vi "filter pipe - complex.vi"(0 "omega  in":dbl[](array[numeric]), 2 "z in":cdb[](array[numeric]), 3 "delta":dbl=0.07, 5 "span":dbl=0.01, 6 "init":bool, 7 "interpolated gamma (kHz)":dbl, 8 "step once":bool, 9 "filter method":T1) -> (10 "center":cdb=0.005233304275841307+0.002092688467219436i, 12 "norm":dbl=0.0018669991905548619, 13 "at right end?":bool=TRUE, 14 "omega out":dbl[](array[numeric])=[2475.05, 2475.14, 2475.23, 2475.32, 2475.41, 2475.5, 2475.59, 2475.68, 2475.77, 2475.86, 2475.95, 2476.04, 2476.13, 2476.22, 2476.31, 2476.4, 2476.49, 2476.58, 2476.67, 2476.76, 2476.85, 2476.94, 2477.03, 2477.12, 2477.21, 2477.3, 2477.39, 2477.48, 2477.57, 2477.66, 2477.75, 2477.84, 2477.93, 2478.02, 2478.11, 2478.2, 2478.29, 2478.38, 2478.47, 2478.56, 2478.65, 2478.74, 2478.83, 2478.92, 2479.01, 2479.1, 2479.19, 2479.28, 2479.37, 2479.46, 2479.55, 2479.64, 2479.73, 2479.82, 2479.91, 2480.0, 2480.09, 2480.18, 2480.27, 2480.36, 2480.45, 2480.54, 2480.63, 2480.72, 2480.81, 2480.9, 2480.99, 2481.08, 2481.17, 2481.26, 2481.35, 2481.44, 2481.53, 2481.62, 2481.71, 2481.8, 2481.89, 2481.98, 2482.07, 2482.16, 2482.25, 2482.34, 2482.43, 2482.52, 2482.61, 2482.7, 2482.79, 2482.88, 2482.97, 2483.06, 2483.15, 2483.24, 2483.33, 2483.42, 2483.51, 2483.6, 2483.69, 2483.78, 2483.87, 2483.96, 2484.05, 2484.14, 2484.23, 2484.32, 2484.41, 2484.5, 2484.59, 2484.68, 2484.77, 2484.86, 2484.95, 2485.04, 2485.13, 2485.22, 2485.31, 2485.4, 2485.49, 2485.58, 2485.67, 2485.76, 2485.85, 2485.94, 2486.03, 2486.12, 2486.21, 2486.3, 2486.39, 2486.48, 2486.57, 2486.66, 2486.75, 2486.84, 2486.93, 2487.02, 2487.11, 2487.2, 2487.29, 2487.38, 2487.47, 2487.56, 2487.65, 2487.74, 2487.83, 2487.92, 2488.01, 2488.1, 2488.19, 2488.28, 2488.37, 2488.46, 2488.55, 2488.64, 2488.73, 2488.82, 2488.91, 2489.0, 2489.09, 2489.18, 2489.27, 2489.36, 2489.45, 2489.54, 2489.63, 2489.72, 2489.81, 2489.9, 2489.99, 2490.08, 2490.17, 2490.26, 2490.35, 2490.44, 2490.53, 2490.62, 2490.71, 2490.8, 2490.89, 2490.98, 2491.07, 2491.16, 2491.25, 2491.34, 2491.43, 2491.52, 2491.61, 2491.7, 2491.79, 2491.88, 2491.97, 2492.06, 2492.15, 2492.24, 2492.33, 2492.42, 2492.51, 2492.6, 2492.69, 2492.78, 2492.87, 2492.96, 2493.05, 2493.14, 2493.23, 2493.32, 2493.41, 2493.5, 2493.59, 2493.68, 2493.77, 2493.86, 2493.95, 2494.04, 2494.13, 2494.22, 2494.31, 2494.4, 2494.49, 2494.58, 2494.67, 2494.76, 2494.85, 2494.94, 2495.03, 2495.12, 2495.21, 2495.3, 2495.39, 2495.48, 2495.57, 2495.66, 2495.75, 2495.84, 2495.93, 2496.02, 2496.11, 2496.2, 2496.29, 2496.38, 2496.47, 2496.56, 2496.65, 2496.74, 2496.83, 2496.92, 2497.01, 2497.1, 2497.19, 2497.28, 2497.37, 2497.46, 2497.55, 2497.64, 2497.73, 2497.82, 2497.91, 2498.0, 2498.09, 2498.18, 2498.27, 2498.36, 2498.45, 2498.54, 2498.63, 2498.72, 2498.81, 2498.9, 2498.99, 2499.08, 2499.17, 2499.26, 2499.35, 2499.44, 2499.53, 2499.62, 2499.71, 2499.8, 2499.89, 2499.98, 2500.07, 2500.16, 2500.25, 2500.34, 2500.43, 2500.52, 2500.61, 2500.7, 2500.79, 2500.88, 2500.97, 2501.06, 2501.15, 2501.24, 2501.33, 2501.42, 2501.51, 2501.6, 2501.69, 2501.78, 2501.87, 2501.96, 2502.05, 2502.14, 2502.23, 2502.32, 2502.41, 2502.5, 2502.59, 2502.68, 2502.77, 2502.86, 2502.95, 2503.04, 2503.13, 2503.22, 2503.31, 2503.4, 2503.49, 2503.58, 2503.67, 2503.76, 2503.85, 2503.94, 2504.03, 2504.12, 2504.21, 2504.3, 2504.39, 2504.48, 2504.57, 2504.66, 2504.75, 2504.84, 2504.93, 2505.02, 2505.11, 2505.2, 2505.29, 2505.38, 2505.47, 2505.56, 2505.65, 2505.74, 2505.83, 2505.92, 2506.01, 2506.1, 2506.19, 2506.28, 2506.37, 2506.46, 2506.55, 2506.64, 2506.73, 2506.82, 2506.91, 2507.0, 2507.09, 2507.18, 2507.27, 2507.36, 2507.45, 2507.54, 2507.63, 2507.72, 2507.81, 2507.9, 2507.99, 2508.08, 2508.17, 2508.26, 2508.35, 2508.44, 2508.53, 2508.62, 2508.71, 2508.8, 2508.89, 2508.98, 2509.07, 2509.16, 2509.25, 2509.34, 2509.43, 2509.52, 2509.61, 2509.7, 2509.79, 2509.88, 2509.97, 2510.06, 2510.15, 2510.24, 2510.33, 2510.42, 2510.51, 2510.6, 2510.69, 2510.78, 2510.87, 2510.96, 2511.05, 2511.14, 2511.23, 2511.32, 2511.41, 2511.5, 2511.59, 2511.68, 2511.77, 2511.86, 2511.95, 2512.04, 2512.13, 2512.22, 2512.31, 2512.4, 2512.49, 2512.58, 2512.67, 2512.76, 2512.85, 2512.94, 2513.03, 2513.12, 2513.21, 2513.3, 2513.39, 2513.48, 2513.57, 2513.66, 2513.75, 2513.84, 2513.93, 2514.02, 2514.11, 2514.2, 2514.29, 2514.38, 2514.47, 2514.56, 2514.65, 2514.74, 2514.83, 2514.92, 2515.01, 2515.1, 2515.19, 2515.28, 2515.37, 2515.46, 2515.55, 2515.64, 2515.73, 2515.82, 2515.91, 2516.0, 2516.09, 2516.18, 2516.27, 2516.36, 2516.45, 2516.54, 2516.63, 2516.72, 2516.81, 2516.9, 2516.99, 2517.08, 2517.17, 2517.26, 2517.35, 2517.44, 2517.53, 2517.62, 2517.71, 2517.8, 2517.89, 2517.98, 2518.07, 2518.16, 2518.25, 2518.34, 2518.43, 2518.52, 2518.61, 2518.7, 2518.79, 2518.88, 2518.97, 2519.06, 2519.15, 2519.24, 2519.33, 2519.42, 2519.51, 2519.6, 2519.69, 2519.78, 2519.87, 2519.96, 2520.05, 2520.14, 2520.23, 2520.32, 2520.41, 2520.5, 2520.59, 2520.68, 2520.77, 2520.86, 2520.95, 2521.04, 2521.13, 2521.22, 2521.31, 2521.4, 2521.49, 2521.58, 2521.67, 2521.76, 2521.85, 2521.94, 2522.03, 2522.12, 2522.21, 2522.3, 2522.39, 2522.48, 2522.57, 2522.66, 2522.75, 2522.84, 2522.93, 2523.02, 2523.11, 2523.2, 2523.29, 2523.38, 2523.47, 2523.56, 2523.65, 2523.74, 2523.83, 2523.92, 2524.01, 2524.1, 2524.19, 2524.28, 2524.37, 2524.46, 2524.55, 2524.64, 2524.73, 2524.82, 2524.91, 2525.0, 2525.09, 2525.18, 2525.27, 2525.36, 2525.45, 2525.54, 2525.63, 2525.72, 2525.81, 2525.9, 2525.99, 2526.08, 2526.17, 2526.26, 2526.35, 2526.44, 2526.53, 2526.62, 2526.71, 2526.8, 2526.89, 2526.98, 2527.07, 2527.16, 2527.25, 2527.34, 2527.43, 2527.52, 2527.61, 2527.7, 2527.79, 2527.88, 2527.97, 2528.06, 2528.15, 2528.24, 2528.33, 2528.42, 2528.51, 2528.6, 2528.69, 2528.78, 2528.87, 2528.96, 2529.05, 2529.14, 2529.23, 2529.32, 2529.41], 15 "z in out":cdb[](array[numeric])=[0.0035833838692532717+0.002461760501094392i, 0.0035771819918613062+0.002383398826822197i, 0.0035896637358900636+0.0024130108513541115i, 0.0035015501499398196+0.0023945340607163883i, 0.0035873008831075383+0.0024778684725931194i, 0.0035885897129709697+0.0024537360214410358i, 0.0035088707757465133+0.0024641292359750115i, 0.003597217082430608+0.0024340750161693436i, 0.003631720010632346+0.0023785862192928116i, 0.0035745568678300942+0.0024422394362636694i, 0.0035399201630911827+0.0024280274828252144i, 0.0035580606682623604+0.002440398374118043i, 0.003625720812311819+0.0024993156448878443i, 0.0036061845801733778+0.0024315190817099427i, 0.0035582145713593683+0.0024459679384418852i, 0.0036421230436132703+0.002476321755287532i, 0.0035287553100427768+0.0023424752263372945i, 0.0036171591899587107+0.0024145250837663765i, 0.003532561868602024+0.0024591572704326142i, 0.003617891441398917+0.0024402679763692995i, 0.0036290045602513504+0.00241579580006542i, 0.0035493444239111218+0.00238313739070125i, 0.0035972555046684535+0.0024044299122573777i, 0.0036200650959092784+0.002371463271576167i, 0.0035308779717337408+0.00241767414631164i, 0.0036295860411505194+0.002419718849243218i, 0.00362174753114682+0.0024941310084549404i, 0.003571450583738286+0.002397048059956567i, 0.0035875818886430635+0.0023666104860356604i, 0.003566860205338471+0.002429081584103935i, 0.0035699525488675442+0.0024844325543031177i, 0.003476064653744224+0.002383633160705297i, 0.0036232175127809203+0.0024294498032392795i, 0.00363288512712673+0.0024981620304337735i, 0.003538396924363967+0.0023959412028212723i, 0.003571271674315685+0.002447098216273019i, 0.003508919154620533+0.0024530259259026043i, 0.0035849575113782862+0.0025155397453185276i, 0.0036048329234809563+0.0023772432894671462i, 0.0035200144964279696+0.00240796542003325i, 0.003602328067965604+0.002424572275891752i, 0.0034745476516245782+0.002382221112974983i, 0.0035828066578929936+0.0024103228090464482i, 0.003508209137008572+0.0024165559812981477i, 0.003578441967986381+0.002496345352566552i, 0.003640325528288482+0.0024364293033093056i, 0.0035714287753764464+0.0024555592011119174i, 0.003524849174803014+0.0024342593151349856i, 0.0035932963150184863+0.002344267588939546i, 0.0035110362839077466+0.0025242421663906433i, 0.003557255513150884+0.0024298617028996163i, 0.0035296673287069915+0.002361252505724584i, 0.0036325163286586837+0.00243280540320604i, 0.0035319294286353803+0.0024436521133638697i, 0.0035662514801884965+0.002422097711200417i, 0.0036020285215899745+0.0024129770481912055i, 0.0035230276280743935+0.002471111600729994i, 0.003584444460381239+0.0024422631002773316i, 0.003578911929285597+0.002409489547620804i, 0.0035529859560006574+0.0024036240734667856i, 0.0035132435147975437+0.0024054904083619247i, 0.003463131857284522+0.0024405503475789193i, 0.0035672637560924068+0.002443560083858346i, 0.0035523125370005176+0.002366368129371733i, 0.0035076520191292086+0.002418906163306224i, 0.003551664199351211+0.002462329924040328i, 0.003445239735916964+0.00236801376516563i, 0.0034899184188964204+0.0024431139214106303i, 0.003555775647106589+0.002433925663904655i, 0.00358456982149389+0.002394500676721203i, 0.0035855105882482956+0.0024514887734179915i, 0.003490961619807174+0.002359758778193443i, 0.003575085524705776+0.002407285136636773i, 0.003494984478986045+0.0023472883264437612i, 0.00353038270763793+0.002480785742445859i, 0.0035289205163657232+0.002404277705104177i, 0.0035934617145982816+0.0023853197249765253i, 0.0035208916723625376+0.002438126880896989i, 0.003559659196326597+0.0023726754777945117i, 0.0035248771706881525+0.0023927999041865084i, 0.003578111016022166+0.00241046426839324i, 0.00347348416676621+0.002352698556809573i, 0.0035632069271169125+0.0024682307994424446i, 0.0035897383252752944+0.0024105615114982924i, 0.0035610717486355098+0.0024251599236607487i, 0.0035243030783033077+0.0024652360862647458i, 0.0035160113035933114+0.002423037671269478i, 0.0035588597476770524+0.002486697366264302i, 0.0035074438090003683+0.00239134085607491i, 0.003518174703528439+0.0024013709200347024i, 0.0036398643730875795+0.0024272678111350323i, 0.0035008074064160778+0.0023720194595876418i, 0.003516827470707867+0.002448120306554464i, 0.003527739480564925+0.002389676925204653i, 0.0035428498413417092+0.0024644931611026333i, 0.0035472289160750426+0.002401539242261267i, 0.0034585535257575443+0.0023903539401807115i, 0.0035495083814771978+0.0024594963301273363i, 0.003513105043814072+0.002310133918995047i, 0.0034602138724093533+0.0023938751959820723i, 0.003550693438342557+0.002346612822562353i, 0.0034987382755111915+0.0024183107993935105i, 0.003573581890041529+0.0024312854816823178i, 0.003479654372321743+0.0024156204296715503i, 0.00352747853508394+0.002470140829737908i, 0.0035122544030378997+0.0024020022810432662i, 0.003475107385817066+0.002397729372742744i, 0.003558857551111249+0.0024913973330730702i, 0.003494633516901589+0.0023768186147511915i, 0.0034596190161777438+0.0024098468261460324i, 0.00355143728276678+0.002322685909100719i, 0.0034708038416920357+0.002429720597385881i, 0.0035037363223939873+0.002451687288317314i, 0.0034956670407026748+0.002372372382178163i, 0.00351113962457242+0.00232323615154957i, 0.0036210465898300153+0.0023834065665714874i, 0.0034975813347267134+0.0023707285810012544i, 0.003514534808645119+0.0023141060324875905i, 0.0035101947703328642+0.002371746120911647i, 0.0034948154899522186+0.0024071024892826313i, 0.0035314751193487284+0.0024235702438064437i, 0.0034677264530420236+0.0023816355176092614i, 0.0035771961236646887+0.0024076893245014224i, 0.0034796189752358546+0.0023209608109559954i, 0.003513251068011808+0.0023907716223097973i, 0.003569326465865384+0.0023886350847090107i, 0.003551974765683957+0.0023796640722348323i, 0.0035080514916192036+0.0023941754660634527i, 0.003484926293668462+0.00231362185533568i, 0.003535211734648734+0.0024050911722595576i, 0.003514987019535619+0.002415959021674241i, 0.0034235890400830414+0.002375631665750588i, 0.0035216639872848+0.0024059040699407398i, 0.0035598915934478754+0.0023663060509351848i, 0.003465427757074372+0.0023383016346386638i, 0.0035276676327022074+0.002332943048272689i, 0.0034422920259387143+0.002349255722960841i, 0.003659840365676227+0.0024070771222320492i, 0.00352624120205378+0.0023103613573044676i, 0.0034588322047578424+0.0023181385790425127i, 0.0035320691029944494+0.0023493092722126456i, 0.0034634662834353413+0.0022926632098579217i, 0.0034889741661585025+0.002382789259467554i, 0.003501069018055188+0.002317901187173858i, 0.0035608795786062123+0.002432557462658446i, 0.0035981890150610196+0.0023361511072360745i, 0.0035227461533919716+0.002344200679224383i, 0.003478178948055545+0.002325184691917999i, 0.0035164872988836583+0.002286116276938515i, 0.003473704407306111+0.002361537640465988i, 0.003552999693395793+0.002335307900326911i, 0.003569561601196032+0.0023659283638241815i, 0.003506002944335002+0.002355817292261747i, 0.003454558431294856+0.002285250434555848i, 0.0036009691145117355+0.002400038934350438i, 0.003467799793673231+0.002336977772979238i, 0.0035586987868674804+0.0022901332320088156i, 0.003568996542700907+0.002333927984249821i, 0.00353813312895247+0.002359668666377636i, 0.003490476090172063+0.002309350991735181i, 0.00352400760763747+0.002329493331797924i, 0.0034463629133157417+0.0023980086128158455i, 0.003535944486126863+0.0024098847747389333i, 0.003557585232599259+0.0023253813452374155i, 0.003571922735920167+0.002422120508457419i, 0.003599966742411332+0.002372732831203898i, 0.003463785224112697+0.002278940673152451i, 0.0034730885706140855+0.002344963600576924i, 0.003505826208382468+0.002359438225862591i, 0.003554322351787642+0.002378191702847825i, 0.003540606126685806+0.0022665507153243492i, 0.00352439286200174+0.0023083330255789414i, 0.0035425444715341935+0.0023670989464567964i, 0.003525622677322043+0.0023382397799141543i, 0.003450636181455629+0.002337118080223388i, 0.0035535402261027134+0.0023314507561510954i, 0.0035792482639411334+0.0023005886295082915i, 0.0035038073247337966+0.002377532544682845i, 0.003528250851607436+0.002298695337920534i, 0.0034838387402360334+0.0023609771360568075i, 0.0034677134358967803+0.0023530426970301958i, 0.0034538269632342533+0.0022708760514073404i, 0.0035354434170829538+0.0023659030754422474i, 0.003588388050736515+0.0023256474670448105i, 0.0035570496027911547+0.0022968149530061023i, 0.0035631120994351066+0.0023102460877339813i, 0.0034446964053939247+0.0023251667507494275i, 0.003581549886958441+0.0023270975147601384i, 0.003558229006462881+0.002256308728031i, 0.0036153564826052454+0.0022819116076532677i, 0.0035698330521307833+0.0023404647043887526i, 0.003557495445685924+0.0021780687906942913i, 0.0035636889137244886+0.002316360143524437i, 0.0035489418247209885+0.0023338911092159157i, 0.0035865936588108916+0.002347201701916542i, 0.003627680277618043+0.002356420764075811i, 0.0035613345052961055+0.0023279985711012925i, 0.0035551999490118927+0.0023350304560901996i, 0.0035907594918857446+0.0023443901240043285i, 0.0034842567382050013+0.0023281743146581378i, 0.0035383427585167077+0.0023472370934859415i, 0.0036090418008660175+0.0022936216813067107i, 0.0035659376898121782+0.00229290291449918i, 0.00352852001705523+0.0022321078053527117i, 0.0035385893524616597+0.0023205455250510736i, 0.0035149970845584784+0.002290337988789042i, 0.0035452937905108926+0.0022792731981642667i, 0.0035599762393293383+0.0022722141868139873i, 0.0035974590595691937+0.0022630875698926444i, 0.0035317566215972316+0.002258735740562212i, 0.003623083174196148+0.0022550653820463764i, 0.0034919286241330036+0.0023056564951337405i, 0.0034693544353237423+0.002341918762057366i, 0.003539476096330802+0.0022151206516599618i, 0.003517617456150341+0.0023196403838069103i, 0.0035822253907969266+0.002303355416174614i, 0.0035378594588336802+0.002158461800458728i, 0.0035088739847597404+0.002316903169197293i, 0.0035834492449240327+0.002338588471356567i, 0.003536536501426079+0.002237279578351037i, 0.0035580853179553677+0.002225762024623049i, 0.0035794887300176176+0.002290589134302724i, 0.003534894770747136+0.002240050534634707i, 0.0036168316737561143+0.0022293367957941356i, 0.003545455375004854+0.0022621350991252156i, 0.0035961876580183016+0.0023301363368508706i, 0.0035729011551604043+0.0022578370543411687i, 0.003559383466164925+0.002255017689957344i, 0.003572984818131717+0.002255315280949931i, 0.0034787854966874393+0.0023216479259984407i, 0.0035949990471021613+0.0023316959144856248i, 0.0035439175006579207+0.0022095875999111453i, 0.003634023139638367+0.002280059495010875i, 0.003586620804902628+0.0023314411084844125i, 0.0035512111777878967+0.0021641612807103226i, 0.0035966175991988215+0.0022622170910395565i, 0.0035865579113099105+0.0021920729784451094i, 0.0036038210771126102+0.002350369977296614i, 0.0036202828789139475+0.0022821148347209616i, 0.003560732360218436+0.002231977509136151i, 0.0035800117922703484+0.002274446351825621i, 0.0035815565105048863+0.0022374872044252578i, 0.0034983402022781902+0.0022305001720500967i, 0.003518818772949233+0.0023401819725400765i, 0.0035699434258511164+0.002349870901262641i, 0.0036439809547703984+0.002267738007340193i, 0.003599468955906992+0.002272859433851576i, 0.003586147637090909+0.002221368238719125i, 0.003613141776701759+0.0022350101562219836i, 0.0035389080427422085+0.0022817793735227187i, 0.0036369038859467013+0.002204530750113422i, 0.0036809645245053555+0.002194426495664775i, 0.0035248720150957455+0.002268690508665336i, 0.0035359807003050763+0.0022255409098568173i, 0.003578056769813253+0.0022884549893426053i, 0.0036110136421018766+0.0022860579273265833i, 0.0035577391275943716+0.002192568027539671i, 0.0036690257277242023+0.0022822388549313547i, 0.003590655471771331+0.0022718474291093934i, 0.0035351068749983005+0.0022096698228379094i, 0.003555789992897444+0.0022938249781770535i, 0.0036198486461379836+0.002207561728496037i, 0.0035926817617155465+0.0022648981141411926i, 0.0036047544924269564+0.002276490438331893i, 0.0035684695813374876+0.0022184590608706964i, 0.003664626266777789+0.002274272578403101i, 0.0035767766497745404+0.0022211446915538745i, 0.0035192532582404845+0.002220796515518189i, 0.003603533155892141+0.0022710350171398852i, 0.003592194915557065+0.0022747277890780306i, 0.0035637022777857386+0.002287589080353134i, 0.0035635670617794905+0.002251607690910359i, 0.003569445701849914+0.002270659553025046i, 0.0036155590827801416+0.002214628868240139i, 0.0034776502347340647+0.002293610092241637i, 0.003543262868696438+0.00231873678594743i, 0.0036389579707786154+0.0022981407339196526i, 0.003577968719193967+0.002232959740098127i, 0.00357353983574272+0.0021742751245045844i, 0.0035128323770260974+0.002209615611307996i, 0.0036088778358281354+0.0022355792361042235i, 0.003582901589164308+0.0022058237286057994i, 0.0036257412099211803+0.0022623733488560034i, 0.0035821258733787806+0.002177272383149605i, 0.003510642931628778+0.002123870480808119i, 0.0035821617241556286+0.0022224362781172627i, 0.003566003401090125+0.002172806735876051i, 0.0035425248618595226+0.002233769991666564i, 0.0036252577664606625+0.0021925451812780097i, 0.003543870751299752+0.0021287701191670667i, 0.0035533293124373464+0.002196398599640853i, 0.0034990126868103665+0.002087830449609492i, 0.003478227374012928+0.0021907025297103707i, 0.003576378375786082+0.002189160934231285i, 0.003492713216935883+0.002164187254120317i, 0.0035510876242912204+0.002181571972376035i, 0.0035206962144764763+0.002110792502252038i, 0.0034813792423866053+0.002103168437224719i, 0.0035688484527795555+0.00204169351547086i, 0.0034592506599694464+0.002096100415609896i, 0.003543217915242846+0.0021662462599298616i, 0.003623123907990784+0.0020268068417267854i, 0.003476643205739687+0.002113910967396962i, 0.0035076341540757334+0.001991261890178615i, 0.0034981803649824918+0.0020840188999582104i, 0.0034606116882584443+0.0020984474581436643i, 0.0034526570429250867+0.001971778912887303i, 0.00349117049441251+0.001995528919514914i, 0.00351179423295713+0.0020196565189796174i, 0.0035119575726532655+0.0019250963537095728i, 0.003433908168342944+0.0019471930739036786i, 0.003422290334470139+0.0018981328016960872i, 0.0034467251049947263+0.001920114507026482i, 0.0034940327967724924+0.0018241309688785516i, 0.0034046416592064524+0.0017479287842611i, 0.003510582434397141+0.0017523636697467503i, 0.003377451300798974+0.0015737217661158495i, 0.003366305085286445+0.0015791833070148142i, 0.003407275726796194+0.0013939125375917107i, 0.0034324044111918+0.0013799224308392404i, 0.0035046357751586077+0.0011791003090811114i, 0.003494602137659145+0.0008518891775068626i, 0.004107292740171204+0.00031669188883613075i, 0.005591741172957749+0.00027393804145127134i, 0.007003031271413257+0.0016339998480635787i, 0.007100303466396169+0.002538127010719567i, 0.0069845033664730025+0.0030550658922751986i, 0.0065897281685950715+0.003397412288409941i, 0.006381102573979224+0.003579172098049876i, 0.006044016406575065+0.0037151359108318215i, 0.005882853510310459+0.0038424641367043127i, 0.0056675754071719535+0.003886563619398313i, 0.00547634520808543+0.0039114388929876i, 0.005327015202010923+0.0038973637277423907i, 0.005139754928753836+0.003796880422852963i, 0.005088188574995865+0.0038220034980205523i, 0.004865766799647193+0.003841130421587106i, 0.004760394088792931+0.003808200082403759i, 0.004615035019456415+0.003702028042457962i, 0.004494928416393764+0.0037136448843374265i, 0.0044584837943632315+0.0038060333100996464i, 0.004241396556668126+0.0036935873417961226i, 0.0042348184713294264+0.003673605149282513i, 0.004195958321922506+0.0035976170275514876i, 0.004124978282698656+0.0035795566550530004i, 0.004132829358493748+0.0035980131872013045i, 0.0040850135623205506+0.0035543461922550243i, 0.004067922558419008+0.0034621245596995172i, 0.004036355420985074+0.003405592921952012i, 0.003928714859908454+0.003391847899602509i, 0.004038319806997925+0.0033805146140530695i, 0.0040208767337669106+0.0033482462799318494i, 0.0038712744979886326+0.003303971321544937i, 0.003969232698420801+0.0032418064872277354i, 0.0038844303767070192+0.0032647750570230765i, 0.0038984043325254723+0.003216004607264936i, 0.003861053267164117+0.0031392317468127927i, 0.0038491394787255944+0.0032044182084920436i, 0.003923299007449422+0.0032031361149841334i, 0.003814605943745064+0.0030932142424365504i, 0.0038487062900693456+0.0031054273621109888i, 0.0038636014850669097+0.003078168173311227i, 0.0038675832214925187+0.003169649663794178i, 0.0038255106579587446+0.00304656886289302i, 0.0037684367340572373+0.003089003666186492i, 0.0038900362933870997+0.0030201045602147297i, 0.003788008514618488+0.0029518881713562657i, 0.0038080963674504286+0.0030222606222834i, 0.0037834217470294196+0.0029869063025990887i, 0.003711013353839813+0.0029907252895459086i, 0.0037255384344122436+0.0029993746748589595i, 0.003666612850703235+0.0029199692412370964i, 0.0036960008624753863+0.002902027308743146i, 0.0037805962978366423+0.0029420687407293276i, 0.0036124349472243635+0.002929986563902275i, 0.0037236360432696316+0.0030102978687088777i, 0.003724023945304685+0.002908898868908707i, 0.0037276613225675093+0.002933293660183733i, 0.003738721152769735+0.002824153275652542i, 0.003687724996401387+0.002869296414638172i, 0.003714560092973169+0.002941154406626834i, 0.0036700279762121417+0.0028606567957325476i, 0.003685810781908494+0.0028970934677133207i, 0.0037745807533508236+0.002898912846243093i, 0.0035960119111983304+0.0027680318284700133i, 0.0036851149473838747+0.002857035032756466i, 0.00360930637526208+0.0028622017097815174i, 0.003669364867234275+0.0028432447367854976i, 0.003768913909328986+0.002831692341251701i, 0.0036534241532698557+0.0027678157881063548i, 0.0037167533276181164+0.0028399723947723507i, 0.0036081078789520758+0.0027470477386512954i, 0.003651094333101398+0.002731573476561886i, 0.003609863299651067+0.0027758808405126266i, 0.0036629144286300097+0.002850381613332309i, 0.003776803096143856+0.0028576113995960354i, 0.0036720584427993863+0.0027651251383553274i, 0.0037547045636355273+0.0027864422078050267i, 0.0036966351651544892+0.0027652823867708575i, 0.003614923529720698+0.002797262614667328i, 0.0036781876862671996+0.002797801073794114i, 0.0036767083481865173+0.0027819892677776402i, 0.003683784344350028+0.0027776871047189284i, 0.003636547190804756+0.002731590075530915i, 0.0036728074808963142+0.0028303680671647995i, 0.00364679379076216+0.0028574019418408283i, 0.0036321001326139204+0.002730742757398695i, 0.003706836087900403+0.0028026187949829013i, 0.003754241548081857+0.0028466157815220466i, 0.003612925716150658+0.002718256171730161i, 0.003644798458003874+0.002750276700162601i, 0.003693164777103008+0.0027982441779361633i, 0.0036940341736720864+0.002824109367571825i, 0.00367515761985943+0.0027518466129067957i, 0.0036549137201372277+0.0027300978457017785i, 0.0037069867237176663+0.00281823311881345i, 0.0036524939336342256+0.002713470147532589i, 0.0036010433993365815+0.0027669613769411303i, 0.0036863269528776043+0.0028225879566892284i, 0.003638718857455406+0.0027117516625715155i, 0.00371418568888802+0.002805978633046487i, 0.0036386709025835453+0.002736862408098532i, 0.003694503290361583+0.0028207231643669235i, 0.0037405549563709387+0.002752461072435501i, 0.0036152800505250544+0.0027190712000436036i, 0.003661423030053704+0.0027336025783764118i, 0.003663389421377418+0.0027684601725113654i, 0.0036951200918362557+0.0027968964767043905i, 0.0036513822699309985+0.0028052541948020426i, 0.0035935302709030133+0.0027540026840236803i, 0.0036603141855145803+0.002782578287736294i, 0.003634206899839832+0.002666523625078767i, 0.0036199060675739026+0.0027452466843605546i, 0.0036216274536002265+0.0027717665058503735i, 0.0036265974054589295+0.0026707503654881896i, 0.003657392196092407+0.0027894282004601754i, 0.0036513527741112318+0.002816983239752639i, 0.0035901020192870563+0.002850209489036475i, 0.00366305904393251+0.002780761135794501i, 0.0035556175680344928+0.002712565224680057i, 0.0036212625000934676+0.0028161773666271084i, 0.0035892185995407885+0.002789925988843793i, 0.003531590955709578+0.0027442509499915977i, 0.0036815058087588015+0.002766098993288713i, 0.003548670832270113+0.0027916064153118625i, 0.0036402506827426795+0.0027653460953164506i, 0.003605596804188133+0.0027380823902546756i, 0.003562110316533151+0.0027405127364629397i, 0.0036415355589932063+0.002646039350233067i, 0.003558595343438631+0.0027060026210251045i, 0.003593136358016868+0.002843810336925084i, 0.003661234502901094+0.002685213325303766i, 0.0035618563735645018+0.0027276782190879013i, 0.0035869193366032887+0.002714046938670368i, 0.003628593918857194+0.0027956963527716538i, 0.003642798309201599+0.002843479831704364i, 0.0035192160404864544+0.00270467305757129i, 0.0035872110056492214+0.002764037053843666i, 0.0036553515891809543+0.0028130188312029346i, 0.0035822323217940045+0.002677164988470653i, 0.0034744616418806392+0.0027582329404408088i, 0.003570136395949138+0.002708133986929033i, 0.0036175829855993706+0.0028112663955769395i, 0.003627828493584409+0.002754399243884811i, 0.003525403770543067+0.002746714088169368i, 0.0036025796973760808+0.00272416212053133i, 0.0035672929146545987+0.0025929508090846783i, 0.0035342832860096526+0.002736408470228262i, 0.0035326213837791128+0.002747898565893272i, 0.0035815910380366978+0.002637262639948765i, 0.0036333889473371124+0.0027471708718967876i, 0.0035850178692254228+0.0027234639668888496i, 0.0035614372018910536+0.0028081247185347724i, 0.003617064013728365+0.0026991588084761837i, 0.003497493372060167+0.002721696749611016i, 0.0035812851855931134+0.002758979433316858i, 0.003557183352009418+0.002691047183462221i, 0.003519731403374078+0.002753088279725155i, 0.0034794952203778297+0.0026536098177210293i, 0.0035221726995946115+0.002685397169971937i, 0.0035696456508317698+0.0027987968539483436i, 0.0035758402998134564+0.0026967610554166272i, 0.0036247276878605705+0.0027835422141590984i, 0.0035462724084365993+0.0027244563095927656i, 0.0035219975311388163+0.0026866695248334888i, 0.0035075207069964255+0.0026876073340291414i, 0.0035528115969558566+0.0026911428197944564i, 0.003554631665044646+0.002736063378757549i, 0.003589495843449941+0.0026507165463976762i, 0.0034760464380063924+0.0026975786274386865i, 0.0035983716672891393+0.0027227420559481647i, 0.0035075681500883037+0.00266883892094949i, 0.003558114896943232+0.002686118167034142i, 0.0035650242287143625+0.0027182458201337727i, 0.0035248842604361837+0.002761875756713414i, 0.0035881126376611115+0.0027632349514284983i, 0.003498272700750322+0.0027314811151279185i, 0.003519529713611601+0.002664798817269026i, 0.0036222905984739213+0.002681884334024452i, 0.0034347747822203786+0.002723024041897357i, 0.0035902204878682734+0.002734221287881907i, 0.0035421892231463086+0.0026735228077247783i, 0.0035013157558732686+0.002756961237349652i, 0.0035799432413238996+0.002591647341865101i, 0.003531356819538718+0.002707567059226137i, 0.003476985648833612+0.002753151340443741i, 0.003502725576008179+0.0026272988228648844i, 0.0034963514969285434+0.002671448421869216i, 0.003542632868123115+0.0026756707356399446i, 0.0034794852220537105+0.00263835012818776i, 0.003488121696013973+0.0026854988574807827i, 0.0035522106794337698+0.0027192101034773097i, 0.003512171129760311+0.002745883928530569i, 0.0035636538380049007+0.002633065820595081i, 0.00349060586133306+0.002616201961072789i, 0.0035808550288741582+0.0027386932040076952i, 0.0034615341449835036+0.0026259374182983973i, 0.00350728569117591+0.0027020979920341632i, 0.0035259259548032587+0.0027526976356581287i, 0.0035317732186492747+0.002619784404628498i, 0.003499572004018449+0.0026280314808071856i, 0.003466201293135228+0.0026846593682146504i, 0.0034771498039128175+0.002663812079370079i, 0.0034907683439742714+0.0026431371793222327i, 0.003521953598032527+0.0026903036449827753i, 0.0034705052680323967+0.002643484682117665i, 0.0035466776179560434+0.0026442372181035524i, 0.003511637214443899+0.002705380885897081i, 0.003440762836422384+0.002669894435310876i, 0.003490099931821212+0.002648301740701297i, 0.003600026859350433+0.002706351413384413i, 0.003446038939295179+0.002590147256245752i, 0.003501756855027542+0.0026910753646426206i, 0.0035385548338487385+0.0026580541446530304i, 0.003380787156969207+0.002695142457063621i, 0.00353364270515508+0.002628423291326872i, 0.0034450134817139134+0.002686529456056793i, 0.0034923132058637773+0.0027088206442244943i, 0.003575556435152152+0.0026149053833669765i, 0.0034824187147572197+0.0025784028253325745i, 0.0035516389004199953+0.0027049813042750626i, 0.003417228740783448+0.0025595276626144007i, 0.003537003063301354+0.00265324336160095i, 0.0035433075306440407+0.002688588221559363i, 0.0035281049866119794+0.002679880483133983i, 0.0035543679648542066+0.0026700981383876382i, 0.0034810110189535037+0.00270475786995446i, 0.003515807898522025+0.002663042582031155i, 0.0034976931275251862+0.002621461307019962i, 0.0034677590390772305+0.002621233893641133i, 0.0035351597278527624+0.002647660593014822i, 0.003578107988508747+0.0026955732981916282i, 0.003520063573353197+0.002675686917127404i, 0.003528134314337787+0.0025892338799367765i, 0.003460791951478829+0.002671408846279301i, 0.003549002096309522+0.002699466480970137i, 0.003436442621164269+0.0026222809501696533i, 0.0035104757557234243+0.002735024689158493i, 0.0035152286194139104+0.002629999112868711i, 0.003444997885725096+0.0026427258923059156i, 0.0035730826166120505+0.0026563185686777156i, 0.0034488934577342873+0.0026501513515514276i, 0.00349723775694925+0.002679095825335297i, 0.0035209325561349598+0.00266141101027317i, 0.0035236166703602576+0.0026034830404942735i, 0.0036161015782167224+0.0027380901755947175i, 0.003466564743252701+0.0025908875369632335i, 0.0034742251829237626+0.0026554891661408845i, 0.00359707895392126+0.002661867849077778i, 0.003549144244508848+0.002675091016731897i, 0.0035413861721946454+0.002597931501181818i, 0.0034396875752807313+0.0026579070768906103i, 0.003519483957027262+0.0026615917366867026i, 0.003584161467316904+0.002556938765942769i, 0.0034153262596669136+0.002624844851770148i, 0.0035860865478413422+0.002698027555006517i, 0.0035988115108080247+0.002676446749069018i, 0.0035001030870069096+0.002680935392055029i, 0.003432201418239093+0.0025860399894193937i, 0.0034741897701897582+0.002684655450436008i, 0.003530747312368005+0.002653721964277347i, 0.0034725613583156682+0.002600804729528433i, 0.0035805327881641928+0.0026964145222213463i, 0.003591939746901675+0.0026556851806239937i, 0.0034174467097082073+0.0026093556578404217i, 0.0035273325752762075+0.002598827030333705i, 0.003536529673819471+0.0026381009404710487i, 0.0035131456022649736+0.002691273333639735i, 0.0034726603486369763+0.002659426758453685i, 0.00348245389235732+0.002654942672375425i, 0.0035715733111946566+0.0026668436210372944i, 0.003438375032567403+0.0026368788009169825i, 0.003458264165765576+0.002624507555945854i, 0.003473813192862017+0.0026789313165182078i, 0.003455032360677824+0.0026442690592960957i, 0.0035884370632634564+0.002651089232930503i, 0.0034540902785073504+0.0026282376206999115i, 0.003535149369835089+0.0026726425579308775i, 0.0035490234515934724+0.0026193828773884045i, 0.0034323348053194504+0.002612578278663595i, 0.0035461284086343798+0.0026994133340041866i, 0.0034600229224960363+0.0026548192944036877i, 0.0034680318494269297+0.00260297441698279i, 0.0034859999557086264+0.002568839203323468i, 0.0034805717726064537+0.00265356622902995i], 16 "z out":cdb[](array[numeric])=[0.0035625870091985437+0.002422625096112168i, 0.0035688503454743307+0.002439827730478175i, 0.0035799803322629988+0.002426914493562038i, 0.0035838407509538057+0.0024283350914563974i, 0.0035856030846732785+0.002430186859177575i, 0.003587569380969158+0.0024340152276324033i, 0.0035843086479959525+0.0024329607079772602i, 0.0035835164661516938+0.0024313766433830836i, 0.0035850008675947917+0.0024319575795035096i, 0.0035837626329120837+0.0024353591426519625i, 0.0035811679175952703+0.0024366015549562832i, 0.0035784219376709748+0.0024402667871356496i, 0.0035753719096975776+0.002443111477544122i, 0.0035727480013135436+0.0024419832519806685i, 0.003571273109988151+0.0024431939323658262i, 0.003565821664458903+0.0024451027724743755i, 0.003562822105347891+0.0024434299731824595i, 0.0035625604426215906+0.0024427673800409i, 0.00356229877989529+0.00244210478689934i, 0.0035620371171689895+0.00244144219375778i, 0.003561775454442689+0.0024407796006162205i, 0.0035615137917163883+0.0024401170074746605i, 0.0035612521289900877+0.002439454414333101i, 0.0035609904662637876+0.002438791821191541i, 0.0035607288035374874+0.0024381292280499815i, 0.003560467140811187+0.0024374666349084215i, 0.0035602054780848862+0.002436804041766862i, 0.0035599438153585856+0.002436141448625302i, 0.003559682152632285+0.0024354788554837425i, 0.0035594204899059845+0.0024348162623421825i, 0.003559158827179684+0.002434153669200623i, 0.0035588971644533837+0.002433491076059063i, 0.003558635501727083+0.0024328284829175035i, 0.003558373839000783+0.0024321658897759435i, 0.0035581121762744824+0.002431503296634384i, 0.003557850513548182+0.002430840703492824i, 0.0035575888508218812+0.0024301781103512644i, 0.0035573271880955807+0.0024295155172097045i, 0.00355706552536928+0.002428852924068145i, 0.00355680386264298+0.002428190330926585i, 0.0035565421999166793+0.0024275277377850254i, 0.0035562805371903788+0.0024268651446434654i, 0.0035560188744640786+0.002426202551501906i, 0.003555757211737778+0.002425539958360346i, 0.0035554955490114774+0.0024248773652187864i, 0.003555233886285177+0.0024242147720772264i, 0.0035549722235588763+0.002423552178935667i, 0.003554710560832576+0.002422889585794107i, 0.0035544488981062755+0.0024222269926525474i, 0.003554187235379975+0.0024215643995109874i, 0.003553925572653675+0.002420901806369428i, 0.003553663909927374+0.002420239213227868i, 0.0035534022472010736+0.0024195766200863084i, 0.003553140584474773+0.0024189140269447484i, 0.0035528789217484725+0.0024182514338031884i, 0.003552617259022172+0.002417588840661629i, 0.0035523555962958717+0.0024169262475200693i, 0.003552093933569571+0.0024162636543785094i, 0.0035518322708432705+0.0024156010612369494i, 0.0035515706081169704+0.00241493846809539i, 0.00355130894539067+0.0024142758749538303i, 0.0035510472826643692+0.0024136132818122704i, 0.0035507856199380686+0.0024129506886707104i, 0.003550523957211768+0.002412288095529151i, 0.0035502622944854675+0.002411625502387591i, 0.0035500006317591673+0.0024109629092460313i, 0.003549738969032867+0.0024103003161044714i, 0.003549477306306566+0.002409637722962912i, 0.003549215643580266+0.002408975129821352i, 0.0035489539808539654+0.0024083125366797923i, 0.003548692318127665+0.0024076499435382323i, 0.0035484306554013642+0.002406987350396673i, 0.0035481689926750637+0.002406324757255113i, 0.0035479073299487635+0.0024056621641135533i, 0.003547645667222463+0.0024049995709719933i, 0.0035473840044961628+0.002404336977830434i, 0.003547122341769862+0.002403674384688874i, 0.0035468606790435616+0.0024030117915473143i, 0.003546599016317261+0.0024023491984057543i, 0.0035463373535909604+0.0024016866052641948i, 0.00354607569086466+0.002401024012122635i, 0.0035458140281383593+0.0024003614189810753i, 0.003545552365412059+0.0023996988258395153i, 0.0035452907026857585+0.0023990362326979557i, 0.0035450290399594584+0.0023983736395563958i, 0.003544767377233158+0.0023977110464148362i, 0.003544505714506857+0.0023970484532732763i, 0.0035442440517805566+0.0023963858601317167i, 0.003543982389054256+0.0023957232669901568i, 0.003543720726327956+0.0023950606738485972i, 0.003543459063601655+0.0023943980807070372i, 0.0035431974008753547+0.0023937354875654777i, 0.0035429357381490546+0.0023930728944239177i, 0.003542674075422754+0.002392410301282358i, 0.0035424124126964534+0.0023917477081407982i, 0.003542150749970153+0.0023910851149992387i, 0.0035418890872438522+0.0023904225218576787i, 0.0035416274245175516+0.0023897599287161187i, 0.0035413657617912515+0.002389097335574559i, 0.003541104099064951+0.0023884347424329997i, 0.0035408424363386503+0.0023877721492914397i, 0.00354058077361235+0.00238710955614988i, 0.0035407248527083665+0.0023862701744693446i, 0.0035406780052805913+0.0023858055223905557i, 0.0035403792521782104+0.0023848866529570926i, 0.003540557398401449+0.00238451027508162i, 0.0035402008071060216+0.002383577095253203i, 0.003539993309937548+0.002382703968817668i, 0.003540245806751373+0.002381744781275605i, 0.003540263900948342+0.002380884160366024i, 0.0035397789010768255+0.002380269279902875i, 0.003540037767688355+0.0023793285914776594i, 0.0035397918231559753+0.0023787159379305817i, 0.003539342760492389+0.0023782295328771607i, 0.0035389265360938737+0.002376809372141247i, 0.003538492738838126+0.002376252252993808i, 0.003538621549531763+0.0023755421445962404i, 0.003538118111061542+0.0023739434877973553i, 0.0035380134349903046+0.002373802906097663i, 0.00353786420423612+0.0023734257505372714i, 0.0035378829497169904+0.0023723143226700035i, 0.0035376002922833825+0.0023712353766943885i, 0.00353737374030193+0.0023706069500871656i, 0.003537303240597115+0.0023698774095545156i, 0.0035374213041562148+0.002368990440098631i, 0.00353706360898377+0.0023684308445714912i, 0.003537396326021588+0.002367996766465701i, 0.003537133299738949+0.0023671825682282455i, 0.00353683893508461+0.0023659950624354952i, 0.0035368570675222413+0.0023652779442752347i, 0.0035363147763650387+0.002365047738887027i, 0.0035364679965840346+0.0023645675973479755i, 0.0035363445662985743+0.0023631949343717496i, 0.0035371358675332673+0.0023626701428811543i, 0.0035369739572430644+0.002362187622142845i, 0.0035365840463865757+0.0023605166920293375i, 0.003536882856640864+0.0023598418901251755i, 0.003536971396789569+0.002358561067404584i, 0.0035374492570215653+0.0023580629549408904i, 0.003537644357907623+0.0023569136462781135i, 0.0035374384190503642+0.002356175234845338i, 0.0035377406347297646+0.002355506340701442i, 0.003537653440536446+0.0023545681632992812i, 0.003537756619944432+0.0023537988497272806i, 0.0035374422299090007+0.0023534560341462686i, 0.0035377498389208757+0.002353132877149895i, 0.0035380977090296445+0.0023520040068823176i, 0.0035379188096958166+0.0023511908581025135i, 0.0035380042137668965+0.0023500218483658393i, 0.003538452671501436+0.002349025861385597i, 0.00353819038969424+0.002348704051317301i, 0.0035388271874688057+0.0023471180625612067i, 0.0035394664694802618+0.0023459362510815053i, 0.003539439059317983+0.002345466333767387i, 0.0035389722289594543+0.0023444301971151855i, 0.0035392065121368577+0.0023436643244897394i, 0.0035394439281405806+0.0023429904200552203i, 0.003539235702593656+0.002341881792354393i, 0.003539978900751624+0.0023409523152474842i, 0.003540024010459605+0.002340109102141671i, 0.003539811240342784+0.002339105772114113i, 0.0035398296079046923+0.002338562161866363i, 0.0035403679293004287+0.002337567789152545i, 0.0035410087522947417+0.002336698242788286i, 0.003541208704167959+0.0023358738177195076i, 0.003541294869304514+0.0023351248689629524i, 0.003542089137564577+0.0023344085241131444i, 0.003542220731932116+0.002333210666674602i, 0.003542571193281065+0.002332466539561375i, 0.003543137689228242+0.002331617573197806i, 0.003543328114140262+0.0023308321201703564i, 0.0035432335633283764+0.002330303049401082i, 0.0035431338106369156+0.0023293147903658334i, 0.0035435204871514694+0.0023288671045892696i, 0.0035437373108573606+0.0023279031548071117i, 0.0035436341387524873+0.002327633639509896i, 0.0035436962919763344+0.0023268486838228814i, 0.0035442557189842637+0.0023263276739748i, 0.0035441910740509454+0.002325564393995435i, 0.0035444539769206316+0.002324245863226073i, 0.003544218716671544+0.002323424628163435i, 0.003544643410492294+0.00232263952524804i, 0.003544678006805517+0.0023216169742305255i, 0.0035454369747882674+0.0023211631935438353i, 0.003545539290313343+0.0023197160389106415i, 0.003545147340797882+0.0023182740461438027i, 0.0035452602330044037+0.0023172669697461823i, 0.0035454677574130035+0.002315812543349349i, 0.0035455949570138917+0.002314874501869505i, 0.003545939168811464+0.002313418336032799i, 0.003546114471589525+0.0023120960697778506i, 0.0035462863898945603+0.0023110722417143824i, 0.0035455927389847694+0.0023093675576903827i, 0.0035454638860674156+0.002308457000086384i, 0.003545760573561209+0.00230717156014165i, 0.003545575904833474+0.0023060406054006234i, 0.0035456174134914607+0.00230463799058166i, 0.0035454820849638+0.002303177005149015i, 0.003545573314678251+0.0023017313708657812i, 0.0035456736703418914+0.002299637558845471i, 0.0035453882166531104+0.002298543889040694i, 0.0035457882443811293+0.002297405761125871i, 0.0035461608572059417+0.002295781717448223i, 0.0035460336858503896+0.0022942583669610076i, 0.0035457041250836494+0.002292044533164616i, 0.003545779513003054+0.0022903821320498815i, 0.0035454316197350826+0.002288531028629974i, 0.003545116544116847+0.002286360391970822i, 0.0035451781238433067+0.002284332680498435i, 0.0035449411657253968+0.0022819771372091114i, 0.00354501505081026+0.0022796908108091195i, 0.0035448580464249478+0.002277358961365813i, 0.003544198459951312+0.002275197092039048i, 0.0035440533677767285+0.0022726319246253062i, 0.0035439917358835427+0.0022694697877767966i, 0.00354351111774959+0.0022663009655848956i, 0.0035434986894752277+0.002263392910740078i, 0.0035422738476958765+0.0022592801601973704i, 0.003541588092290983+0.0022552577674224486i, 0.0035410306041224163+0.0022505606737665902i, 0.003540622950666575+0.0022455151064020317i, 0.0035406596646636785+0.002239271587736481i, 0.00354046804819428+0.00223127414248953i, 0.003543722881933678+0.0022207396289964706i, 0.0035540531654730976+0.0022098634109922848i, 0.003572081265234354+0.0022063763478523037i, 0.0035904401698712363+0.0022071851552879973i, 0.0036079299287176793+0.002210652281999041i, 0.0036234759838145755+0.0022159155233037442i, 0.003624761919214058+0.002214520600863344i, 0.003625792343897806+0.002212540259210176i, 0.003627365528749319+0.0022107165465313976i, 0.0036285692231568327+0.002209241880145944i, 0.003630078850620531+0.002207850136779489i, 0.003615122915121112+0.0021990375960530386i, 0.0036163976954264035+0.002197698215016473i, 0.003617729027545759+0.002196019107121175i, 0.0036181868899870617+0.002193939973049426i, 0.0036195096760864645+0.002192351213865849i, 0.003620920669601705+0.0021908450603909967i, 0.003602217502409103+0.00218282326568995i, 0.003603099658199955+0.0021809376970949265i, 0.0036041684052611263+0.0021793397754099565i, 0.003604797382963272+0.0021773194728983117i, 0.003605982935195567+0.002175570151986947i, 0.003607387128602013+0.002172779214060266i, 0.0036079456896162326+0.0021702814898839863i, 0.003608917152439218+0.002168302016135497i, 0.0036104326626868926+0.0021659491529197094i, 0.003611267220550441+0.0021639063461924663i, 0.003588884169733501+0.0021577927720796i, 0.0035900360710838276+0.0021554023369395594i, 0.0035907040603513187+0.0021528848247081575i, 0.0035918592701429594+0.0021504204145000438i, 0.0035936517771510057+0.0021481271632352796i, 0.003594119326778623+0.0021453096892502634i, 0.0035946261719768664+0.002142993362101966i, 0.0035958030184319936+0.002140293806584794i, 0.0035959713729800565+0.0021383214441902153i, 0.003569557108412738+0.00213897185326084i, 0.0035695923946830123+0.002135827824267096i, 0.0035692285543541093+0.002132561364495168i, 0.003569182119424985+0.0021292299903918374i, 0.0035700880490618977+0.002125823000691116i, 0.0035698258199099303+0.0021230029217679533i, 0.0035704161529211886+0.0021203573831621875i, 0.0035526869958115506+0.002132868645516283i, 0.003570965636529928+0.0021147902839123165i, 0.0035523560164258125+0.0021277597065098458i, 0.003572419450390771+0.0021083341903799964i, 0.0035531879741292315+0.002121404765624105i, 0.003553691199040588+0.002119073791230589i, 0.003553540553052189+0.0021157313730171133i, 0.0035532183547257574+0.0021128091318771856i, 0.003552747738369849+0.0021102113801046455i, 0.0035458936354283085+0.002124548588540504i, 0.0035520375754291185+0.0021030349992991067i, 0.003545521872965046+0.0021171219789075085i, 0.003552111864697351+0.002095088575816374i, 0.00354392954916202+0.0021109258116408956i, 0.0035427999828177093+0.0021080209618151574i, 0.0035411604354127066+0.002102980019643181i, 0.0035403962176682115+0.0020991344282617953i, 0.0035403027417202342+0.002095539633697904i, 0.0035393465540448843+0.0021042553062870953i, 0.003537961400212195+0.0020841560680566014i, 0.0035367483951148433+0.002095622402991115i, 0.0035348097590437184+0.002075222181547184i, 0.0035332941609380573+0.002087542390870716i, 0.003531413945821079+0.0020813329924452293i, 0.003528879058505537+0.002076166322255621i, 0.0035276852664089878+0.002070559756769113i, 0.0035247859776086545+0.0020774576778666864i, 0.0035231317871338235+0.0020569087501193352i, 0.003519006323367564+0.0020642530770827324i, 0.0035172652295312845+0.002056937619689142i, 0.0035147959173586025+0.002047782092920473i, 0.00351255114841543+0.002038635036020028i, 0.0035108842389118865+0.002028983316526822i, 0.0035072639199511795+0.0020163347276112987i, 0.003505758545454204+0.001989794227302775i, 0.0035010198565802847+0.001995769900098923i, 0.0034958190758545924+0.0019829599591241636i, 0.003492878115765016+0.0019727492237952143i, 0.003488238935994356+0.0019589767149634694i, 0.0034826027627013973+0.0019427704412992928i, 0.0034783159123673575+0.001927299564245782i, 0.0034769273689347+0.001911011743837528i, 0.0034724616998637195+0.001890090392015489i, 0.003467262239573098+0.0018680427519688868i, 0.0034619621712673222+0.0018473051727214385i, 0.0034574441596964896+0.001818243819966927i, 0.0034486864226109465+0.0017882677520074256i, 0.003442459750297909+0.0017541179352794872i, 0.0034387630861745086+0.0017121222528247088i, 0.00344340035386684+0.0016388058687903104i, 0.0034230698013945652+0.0016024531459033246i, 0.0034366907267889078+0.001508188221251121i, 0.0034464767267684106+0.0013671257007145676i, 0.0034496612873088665+0.0013223176911040403i, 0.0034764400425292196+0.0011098615036540973i, 0.003508312971236857+0.0008729540124762158i, 0.004003505366835951+0.00035135624835221156i, 0.005446448201245334+0.00019186413457029298i, 0.007015224327135097+0.0014001972390640508i, 0.0073193064503082675+0.0026141161180456202i, 0.007020015415624015+0.0031195972724585913i, 0.006636224018254199+0.0034265110359800893i, 0.00635007764010221+0.0036059365291323444i, 0.0061015396577520555+0.0037071020763822403i, 0.005878799754674854+0.0038083090807419706i, 0.005671783048105356+0.003870551061438579i, 0.005495510075695435+0.0038939362965433296i, 0.005316033114439092+0.0038589054280012535i, 0.005190239469835224+0.0038384821609113483i, 0.005033415798309496+0.0038321656753858395i, 0.004895500883285887+0.0038197079013270424i, 0.00475610445184947+0.0037736976758237888i, 0.004621137370117735+0.0037418194251118216i, 0.004530918455433998+0.0037577324060730543i, 0.004414139332582437+0.003725897174906098i, 0.004349021755846054+0.003683573420070134i, 0.004282057457066873+0.0036595987597301295i, 0.004243058130876325+0.003624278550829985i, 0.004189349008410379+0.0035848452514438715i, 0.004132829581662659+0.003551058497375868i, 0.004125887975536832+0.0035137620591129196i, 0.004090541642406664+0.003479859694824141i, 0.004054303689620724+0.0034492638848208257i, 0.00402291539948009+0.003412280997705814i, 0.004001095682415176+0.00338083305511472i, 0.00398685197445568+0.003354404755429733i, 0.003967716870320777+0.0033243842478371745i, 0.003958412020907138+0.0033048206494643044i, 0.00394063674640206+0.0032760839576441805i, 0.003930916342756457+0.0032558597434237196i, 0.003919856942414786+0.0032329054391135098i, 0.0039045755802475293+0.0032093573245647383i, 0.003889506766900452+0.0031931297037268713i, 0.0038725481325029157+0.003169449328934831i, 0.0038569673361774828+0.0031448388932269426i, 0.0038451756664663614+0.003130041486974144i, 0.003837285819041418+0.003119180583014472i, 0.0038311153095985577+0.0031039974159714776i, 0.0038196279157010123+0.0030843388079951355i, 0.0038154663513020977+0.0030808436914097357i, 0.00380802490135134+0.0030643395195805866i, 0.0037990162346051353+0.003050900768155551i, 0.0037909324976643363+0.003041158947114624i, 0.0037845104887504893+0.0030264890286161986i, 0.0037818500807272303+0.003018862623047877i, 0.00377302640422651+0.0030030568329154836i, 0.003767084133647707+0.00299498819245826i, 0.0037656781208253486+0.0029875281753712i, 0.003764410549630827+0.0029791377857234912i, 0.003759908044084384+0.0029723333534402274i, 0.00375710810133189+0.0029653349058268007i, 0.00375351852657178+0.002958900819616226i, 0.0037496157613987205+0.0029534027932891197i, 0.003749257205601429+0.0029493765552335103i, 0.003749298681460832+0.002947862879194882i, 0.003747472623490328+0.0029431868024318293i, 0.003745635382417998+0.0029383547411939324i, 0.0037422456213832083+0.002932765730330339i, 0.003740110343124966+0.002928291102223604i, 0.0037384892224267083+0.0029241829218577455i, 0.0037406774950601634+0.00292575929607387i, 0.003738787968320024+0.002921491027332664i, 0.0037372691914901645+0.0029187234935992923i, 0.003734656298792755+0.0029152576145582585i, 0.0037321712862071936+0.0029104210234726993i, 0.0037297320968776217+0.0029061773067045877i, 0.003730747884878853+0.0029106816473009607i, 0.003728172516374503+0.0029072726974745874i, 0.003725618663389812+0.002905239493926145i, 0.0037232013372860383+0.002902260000498734i, 0.0037206295999788457+0.0028998871023651557i, 0.0037179433941660744+0.002896800698684929i, 0.003715689990982847+0.002892560982230627i, 0.003714059179831356+0.002890230009452719i, 0.003711467321429794+0.0028871401849766246i, 0.003711940032664343+0.002890335564103522i, 0.0037103868584477963+0.002888645145918856i, 0.003707217638012632+0.0028857384355729767i, 0.0037053165823798095+0.002883672127489539i, 0.0037031803081765844+0.002881514487168066i, 0.00370125762114856+0.0028778586222162894i, 0.003698535390587881+0.002875725126833942i, 0.0036971229311498466+0.002872836027437025i, 0.0036983079614138622+0.0028752793210363426i, 0.003695895306506089+0.0028732868982385006i, 0.003693541990264217+0.002871070795921578i, 0.003690687001295564+0.002868119250098092i, 0.00368899626845673+0.0028664287291714262i, 0.003687542625064116+0.0028648775449090433i, 0.003685099734093935+0.0028623952297273294i, 0.003683286051446689+0.002860362682458364i, 0.00368122605479984+0.0028578273775632292i, 0.003679504884572229+0.0028556634403635725i, 0.003677948740996124+0.0028536456698568502i, 0.0036763650955602004+0.0028525008050142263i, 0.0036741852680567243+0.0028505213143985787i, 0.0036723219320306325+0.0028486499704411736i, 0.0036709983766397445+0.002846844399731513i, 0.003669378697262484+0.002844702997369602i, 0.003667335711732546+0.002843328136184944i, 0.0036652856049053974+0.0028409693146826797i, 0.0036634288409643527+0.002838762879192221i, 0.003661728855185431+0.002837165240051679i, 0.0036602842285372132+0.0028354490254284587i, 0.003658847418809513+0.0028336292705119052i, 0.0036568374589429128+0.002831692856253836i, 0.003655393158101771+0.0028300601791127165i, 0.0036534509962713787+0.002828119345798426i, 0.0036515652247753935+0.002826189270969426i, 0.003649860145654834+0.002824453477211006i, 0.0036485601790056618+0.0028228440760899296i, 0.003646585193220708+0.002821095950834787i, 0.0036452816783861678+0.002819266821423139i, 0.0036439748750041285+0.0028177607947703384i, 0.0036420232657352935+0.002816149632188507i, 0.0036402336996620103+0.0028149512814484006i, 0.0036391121453762873+0.002812720578327426i, 0.003637552072780926+0.0028109042028872724i, 0.0036365946034344204+0.002809520784088449i, 0.003633338794896165+0.002805052630847634i, 0.0036305610563928834+0.0028006228768451026i, 0.0036273704725145093+0.0027962829563179595i, 0.003624589865660734+0.002791941383813593i, 0.0036217997787635356+0.0027878331613830462i, 0.0036190095240981857+0.0027839978306059307i, 0.0036170848561178667+0.0027803653719703494i, 0.003614851850080103+0.002777034158048962i, 0.0036124063463852194+0.002773757803164207i, 0.0036107248894119946+0.002770253217088192i, 0.003608226217699194+0.0027674706608353835i, 0.003606589434156585+0.0027647218406130275i, 0.0036043090788185875+0.002761813801880098i, 0.003602588921929874+0.002759854711361692i, 0.003600951125959464+0.0027570436011707024i, 0.003598596154086047+0.002754304725073369i, 0.003597422593005055+0.0027521667797923907i, 0.003595448616291688+0.0027499389471637237i, 0.003593651011148659+0.0027479916162975594i, 0.003591956118153282+0.0027455127997795237i, 0.0035904785246233927+0.0027433319471237053i, 0.0035897505995611287+0.0027416365433101347i, 0.003587670013565459+0.0027395200517865543i, 0.003586121669890769+0.0027380643457199285i, 0.0035851062161595185+0.00273630214667159i, 0.003583964586048097+0.0027347788365409756i, 0.0035831329918504335+0.0027328422767522254i, 0.003581710560383311+0.0027311718055013905i, 0.003580981707491795+0.0027299039153538852i, 0.003580442585718136+0.0027281868657311912i, 0.0035786304566435513+0.0027266249674060025i, 0.003578505180216165+0.00272549675258i, 0.003577908489337322+0.0027238707522469225i, 0.003576804437535286+0.0027227575785930508i, 0.0035753353096396314+0.0027210408760159235i, 0.0035740283471956836+0.0027203565811540994i, 0.0035732576151722793+0.0027192961683201477i, 0.0035720595315749584+0.0027176182069587585i, 0.0035716298387044663+0.002716819019050385i, 0.0035711825490205296+0.002715635582828537i, 0.0035694130952146647+0.002714206381736217i, 0.003569068853640023+0.0027133552862921985i, 0.003568341829649417+0.0027122761192691592i, 0.003567861073326771+0.002711444738934666i, 0.003566883222673176+0.0027105419482596157i, 0.0035654754232499856+0.002709672208063736i, 0.0035650819356715657+0.0027091719564183003i, 0.003563700589137289+0.002708170128747912i, 0.003562945852908281+0.0027075536669162003i, 0.0035620635471613395+0.002707290870458703i, 0.003561284266695623+0.002706636758896898i, 0.0035609326161442478+0.002705658249802866i, 0.0035593432184843547+0.002704528078669485i, 0.0035586750395117574+0.0027040720552972556i, 0.0035576792989075517+0.0027032404511362477i, 0.0035563663133494055+0.0027024763491268213i, 0.003556031001436844+0.0027020029876696655i, 0.003554949376725818+0.0027012987214550745i, 0.003553916242438686+0.002700405376123053i, 0.00355300755342564+0.002699602801686702i, 0.0035520988644125928+0.002698800227250351i, 0.003551190175399546+0.0026979976528139996i, 0.0035502814863864994+0.0026971950783776484i, 0.0035493727973734523+0.002696392503941297i, 0.003548464108360406+0.0026955899295049456i, 0.003547555419347359+0.0026947873550685945i, 0.003546646730334312+0.0026939847806322433i, 0.0035457380413212655+0.0026931822061958917i, 0.0035448293523082184+0.0026923796317595405i, 0.003543920663295172+0.0026915770573231893i, 0.003543011974282125+0.002690774482886838i, 0.0035421032852690783+0.002689971908450487i, 0.0035411945962560316+0.0026891693340141357i, 0.0035402859072429845+0.002688366759577784i, 0.0035393772182299383+0.002687564185141433i, 0.003538468529216891+0.0026867616107050817i, 0.0035375598402038444+0.00268595903626873i, 0.0035366511511907978+0.002685156461832379i, 0.0035357424621777506+0.0026843538873960278i, 0.0035348337731647044+0.0026835513129596766i, 0.0035339250841516573+0.0026827487385233254i, 0.0035330163951386106+0.002681946164086974i, 0.003532107706125564+0.0026811435896506226i, 0.0035311990171125168+0.0026803410152142714i, 0.00353029032809947+0.00267953844077792i, 0.0035293816390864234+0.002678735866341569i, 0.0035284729500733767+0.0026779332919052174i, 0.00352756426106033+0.0026771307174688662i, 0.003526655572047283+0.002676328143032515i, 0.003525746883034236+0.002675525568596164i, 0.0035248381940211895+0.0026747229941598127i, 0.003523929505008143+0.002673920419723461i, 0.003523020815995096+0.00267311784528711i, 0.003522112126982049+0.0026723152708507587i, 0.0035212034379690023+0.0026715126964144075i, 0.0035202947489559556+0.002670710121978056i, 0.003519386059942909+0.0026699075475417047i, 0.0035184773709298622+0.0026691049731053535i, 0.003517568681916815+0.0026683023986690023i, 0.0035166599929037684+0.002667499824232651i, 0.0035157513038907217+0.0026666972497962995i, 0.003514842614877675+0.0026658946753599483i, 0.0035139339258646284+0.002665092100923597i, 0.0035130252368515812+0.002664289526487246i, 0.0035121165478385345+0.0026634869520508943i, 0.003511207858825488+0.002662684377614543i, 0.0035102991698124407+0.002661881803178192i, 0.0035093904807993945+0.002661079228741841i, 0.0035084817917863474+0.0026602766543054896i, 0.0035075731027733007+0.0026594740798691384i, 0.003506664413760254+0.002658671505432787i, 0.003505755724747207+0.0026578689309964356i, 0.0035048470357341606+0.0026570663565600844i, 0.0035039383467211135+0.002656263782123733i, 0.0035030296577080668+0.0026554612076873816i, 0.00350212096869502+0.0026546586332510305i, 0.003501212279681973+0.0026538560588146793i, 0.0035003035906689267+0.002653053484378328i, 0.0034993949016558796+0.002652250909941977i, 0.003498486212642833+0.0026514483355056253i, 0.003497577523629786+0.002650645761069274i, 0.003496668834616739+0.002649843186632923i, 0.003495760145603693+0.0026490406121965717i, 0.0034948514565906457+0.00264823803776022i, 0.003493942767577599+0.002647435463323869i, 0.0034930340785645523+0.0026466328888875177i, 0.003492125389551505+0.0026458303144511666i, 0.003491216700538459+0.0026450277400148154i, 0.003490308011525412+0.0026442251655784637i, 0.003489399322512365+0.0026434225911421126i, 0.0034884906334993184+0.0026426200167057614i, 0.0034875819444862713+0.00264181744226941i, 0.003486673255473225+0.0026410148678330586i, 0.003485764566460178+0.0026402122933967074i, 0.003484855877447131+0.002639409718960356i, 0.0034839471884340846+0.002638607144524005i, 0.0034830384994210374+0.002637804570087654i, 0.0034821298104079908+0.0026370019956513022i, 0.003481221121394944+0.002636199421214951i, 0.003480312432381897+0.0026353968467786i, 0.0034794037433688503+0.0026345942723422487i, 0.0034784950543558036+0.002633791697905897i, 0.0034775863653427564+0.002632989123469546i, 0.00347667767632971+0.0026321865490331947i, 0.003475768987316663+0.0026313839745968435i, 0.0034748602983036164+0.0026305814001604923i, 0.0034739516092905697+0.002629778825724141i, 0.0034730429202775226+0.0026289762512877895i, 0.0034721342312644763+0.0026281736768514383i, 0.003471225542251429+0.002627371102415087i, 0.0034703168532383825+0.0026265685279787355i, 0.003469408164225336+0.0026257659535423843i, 0.0034684994752122887+0.002624963379106033i, 0.0034675907861992424+0.002624160804669682i, 0.0034666820971861953+0.0026233582302333308i, 0.0034657734081731486+0.0026225556557969796i, 0.003464864719160102+0.002621753081360628i, 0.003463956030147055+0.002620950506924277i, 0.0034630473411340085+0.0026201479324879256i, 0.005233304275841307+0.002092688467219436i], 19 "tale of three indices -- int -- control out":T2={"left"=403, "center"=604, "right"=604, "right most"=604, "left most"=0, "window"=201, "max win factor"=2, "max win"=2, "min win"=2})   [LabVIEW 2018]
uses:
  tale of three indices -- int -- control.ctl
  filter method control.ctl
  tale of three indices -- selector -- control.ctl
  comparison control.ctl
  command stack.vi
  tale of three indices -- check state.vi
  Q -- check range -- i -- integer.vi
  Q - not nan -- real.vi
  Q - not nan -- integer.vi
panel:
  out "Numeric 2":i32
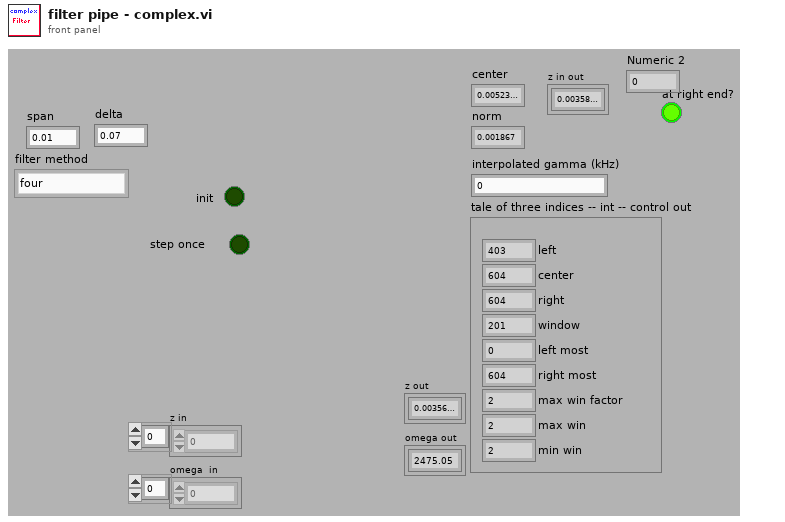
[diagram p1: front panel]
types:
  T1 = typedef "filter method control.ctl" = enum16{"four", "five", "one", "two", "three", "zero", "minus one", "minus two"}
  T2 = typedef "tale of three indices -- int -- control.ctl" = cluster{"left":i32, "center":i32, "right":i32, "right most":i32, "left most":i32, "window":i32, "max win factor":i32, "max win":i32, "min win":i32}
  T3 = typedef "tale of three indices -- selector -- control.ctl" = enum16{"window right", "window left", "balance", "shrink", "grow", "do nothing", "reset", "center right", "center left", "all left", "all right", "right wing shrink", "left wing shrink", "left wing grow", "right wing grow", "skew left", "skew right", "check"}
  T4 = typedef "comparison control.ctl" = enum16{"not a number", "above", "in range", "below"}
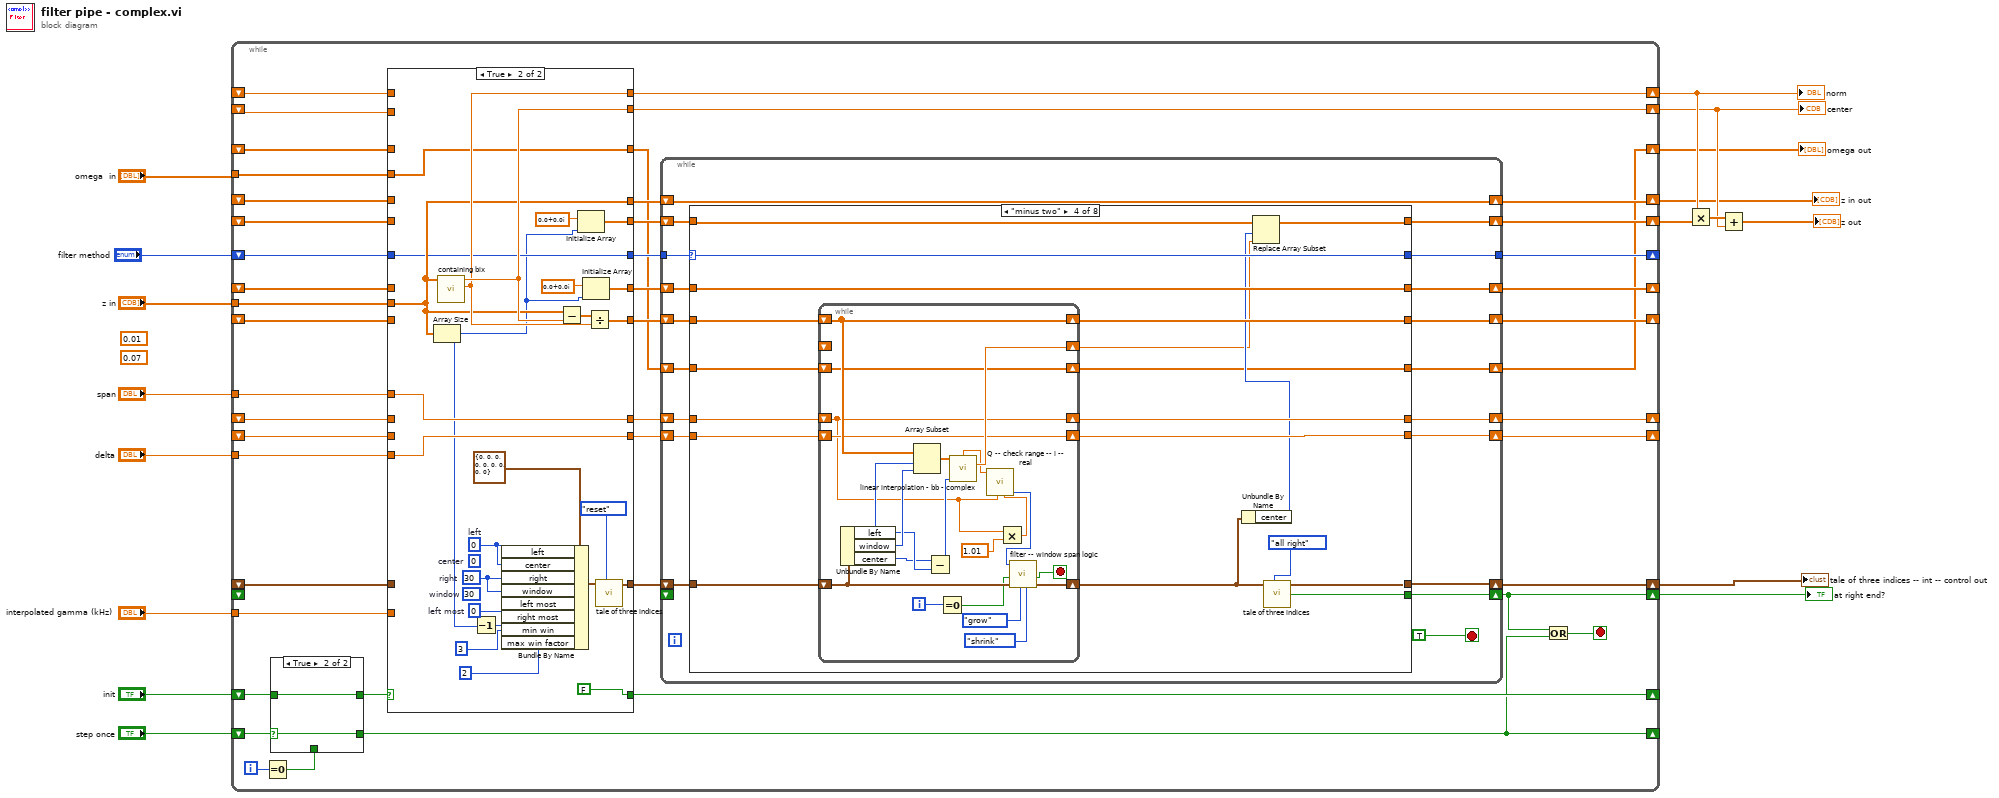
[diagram p0: block diagram]
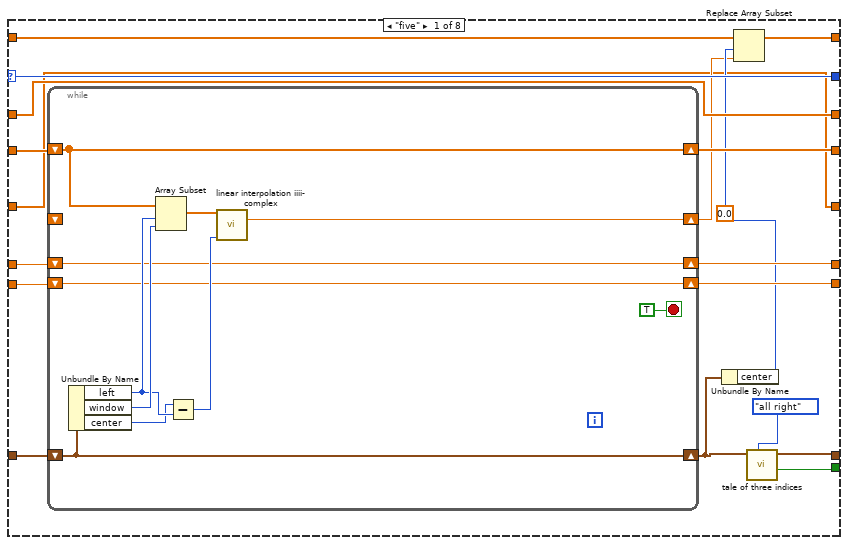
[diagram p4: hidden frame]
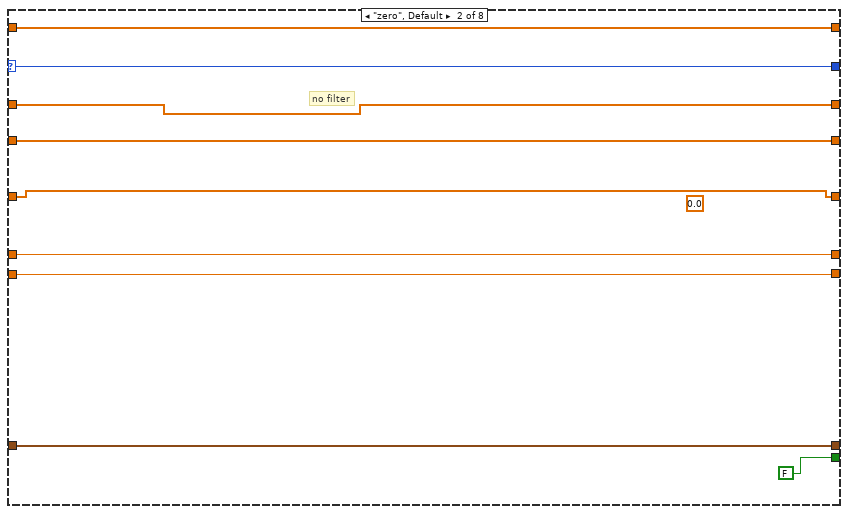
[diagram p5: hidden frame]
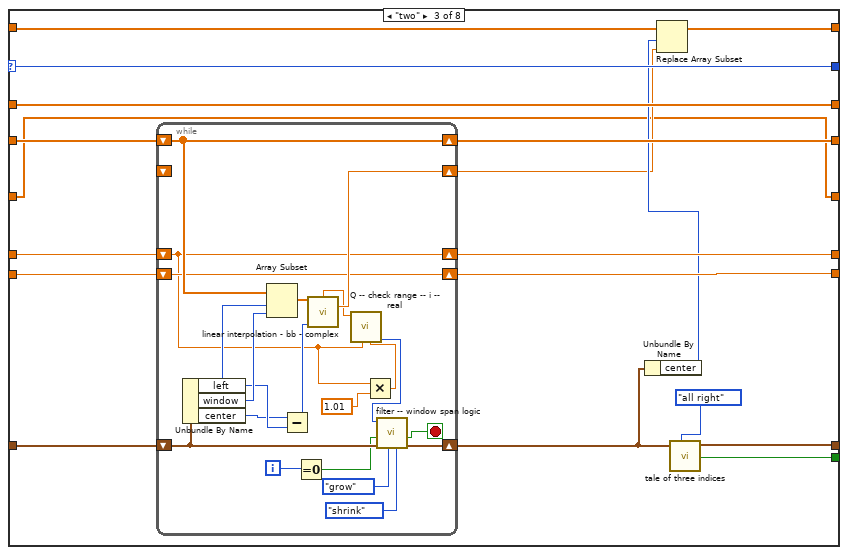
[diagram p6: hidden frame]
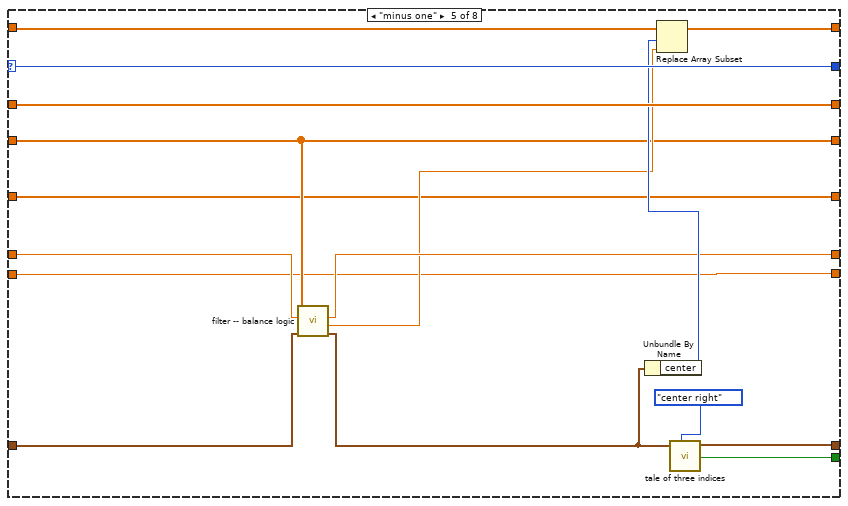
[diagram p7: hidden frame]
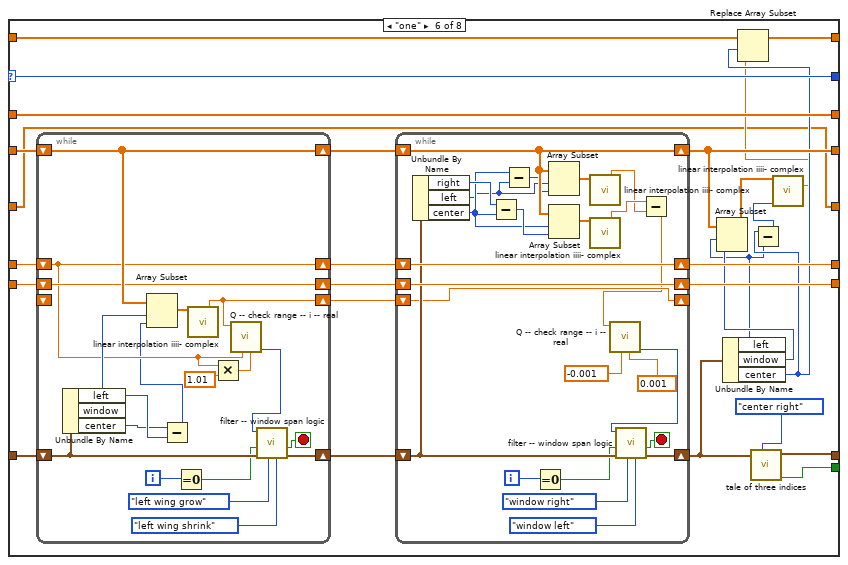
[diagram p8: hidden frame]
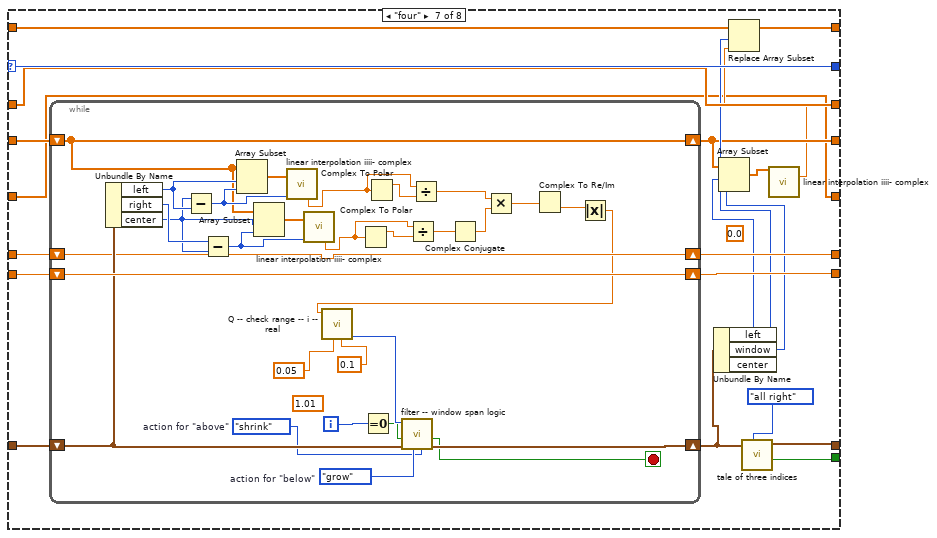
[diagram p9: hidden frame]
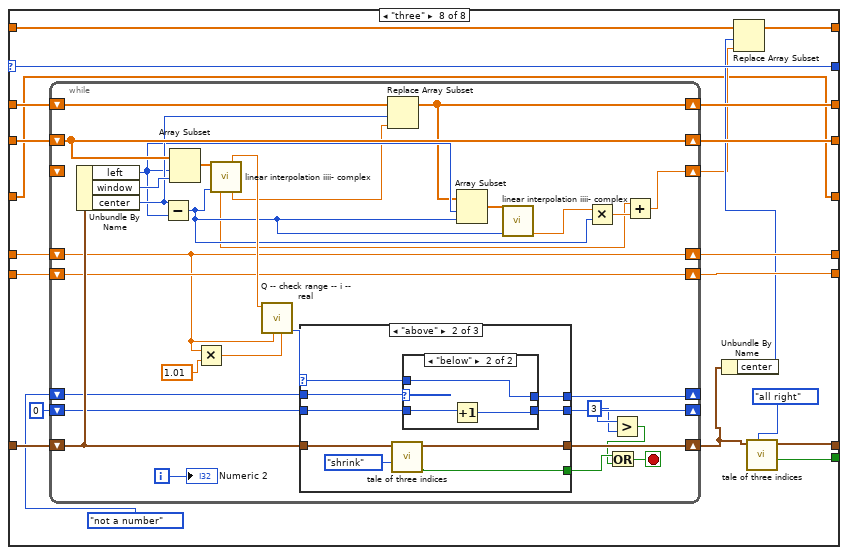
[diagram p10: hidden frame]
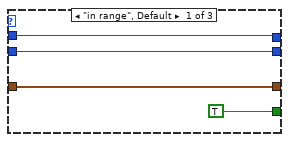
[diagram p11: hidden frame]
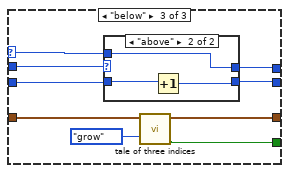
[diagram p13: hidden frame]
diagram:
  (unwired) 0.07
  (unwired) 0.01
  n1 = while {
    tunnel: "z in" -> [w62]
    shift-right: [w41] -> _
    shift-left: _ -> [w59]
    shift-right: [w43] -> w9
    shift-left: _ -> [w58]
    shift-right: [w57] -> w10
    shift-left: _ -> [w55]
    shift-right: [w56] -> w11
    shift-left: _ -> [w54]
    shift-right: [w37] -> w16
    shift-left: _ -> [_]
    shift-right: [w52] -> _
    shift-left: _ -> [w49]
    shift-right: [w51] -> _
    shift-left: _ -> [w47]
    tunnel: "span" -> [w46]
    tunnel: "delta" -> [w53]
    shift-right: [w42] -> w12
    shift-left: _ -> [w44]
    shift-right: [w18] -> w1
    shift-left: _ -> [w40]
    tunnel: "omega  in" -> [w39]
    tunnel: "interpolated gamma (kHz)" -> [w38]
    shift-right: [w36] -> w3
    shift-left: _ -> [w34]
    shift-right: [w27] -> _
    shift-left: "init" -> [w29]
    shift-right: [w26] -> _
    shift-left: "step once" -> [w31]
    shift-right: [w23] -> _
    shift-left: "filter method" -> [w24]
    shift-right: [w21] -> _
    shift-left: _ -> [w20]
    i -> [w33]
    stop <- w32 stop-if-true
    n2 = Equal To 0?(x=w33) -> (x = 0?=w28:bool)
    n3 = case shown="True" w31 {
      selector: w31 -> [w64 w66]
      tunnel: [w64 w66] -> w26
      tunnel: [w63 w65] -> w30
      tunnel: w29 -> [_ w65]
      tunnel: w28 -> [w63 _]
      frame False {
      }
      frame True {
      }
    }
    n4 = case shown="True" w30 {
      selector: w30 -> [w69 _]
      tunnel: w62 -> [_ w87]
      tunnel: [w78 w102] -> w61
      tunnel: [w77 w101] -> w60
      tunnel: [w76 w95] -> w57
      tunnel: [w75 w94] -> w56
      tunnel: w59 -> [w78 _]
      tunnel: w58 -> [w77 _]
      tunnel: w55 -> [w76 _]
      tunnel: w54 -> [w75 _]
      tunnel: [w73 w93] -> w48
      tunnel: w53 -> [_ w93]
      tunnel: [w74 w92] -> w50
      tunnel: w49 -> [w74 _]
      tunnel: w47 -> [w73 _]
      tunnel: w46 -> [_ w92]
      tunnel: [w72 w90] -> w45
      tunnel: w44 -> [w72 _]
      tunnel: w40 -> [w71 _]
      tunnel: [w71 w89] -> w19
      tunnel: w39 -> [_ w89]
      tunnel: w38 -> [_ _]
      tunnel: [w70 w87] -> w35
      tunnel: w34 -> [w70 _]
      tunnel: [w69 FALSE] -> w27
      tunnel: [w68 w85] -> w25
      tunnel: w24 -> [w68 w85]
      tunnel: [w67 w82] -> w22
      tunnel: w20 -> [w67 _]
      frame False {
      }
      frame True {
        w99 = 0  # left most
        (unwired) 30  # window
        w79 = 30  # right
        w98 = 0  # left
        (unwired) 0  # center
        n5 = Array Size(array=w87) -> (size(s)=w83:i32)
        n6 = call "containing bix.vi"("z in"=w87) -> ("norm"=w94:dbl, "center"=w95:cdb)  [unwired: 9 in]
        n7 = Decrement(x=w83) -> (x-1=w88:i32)
        n8 = Bundle By Name(cluster=T2 {"left"=0, "center"=0, "right"=0, "right most"=0, "left most"=0, "window"=0, "max win factor"=0, "max win"=0, "min win"=0} ("tale of three indices"), "left"=w98, "center"=w98, "right"=w79, "window"=w79, "left most"=w99, "right most"=w88, "min win"=3, "max win factor"=2) -> (w97:T2)
        n9 = Subtract(x=w87, y=w95) -> (x-y=w103:cdb[])
        n10 = Initialize Array(cdb 0.0+0.0i, w83) -> (w90:cdb[])
        n11 = Initialize Array(cdb 0.0+0.0i, w83) -> (w82:cdb[])
        n12 = Divide(x=w103, y=w94) -> (x/y=w102:cdb[])
        n13 = call "tale of three indices.vi"("selector"=tale_of_three_indices_--_selector_--_control."reset", "tale of three indices -- int -- control"=w97) -> ("tale of three indices -- int -- control out"=w101:T2)  [unwired: 6 in, 3 out]
      }
    }
    n14 = while {
      shift-right: [w108] -> w43
      shift-left: w60 -> [w121]
      shift-right: [w119] -> w41
      shift-left: w61 -> [w120]
      shift-right: [w109] -> w37
      shift-left: _ -> [_]
      shift-right: [w118] -> w51
      shift-left: w48 -> [w116]
      shift-right: [w117] -> w52
      shift-left: w50 -> [w122]
      shift-right: [w106] -> w42
      shift-left: w45 -> [w107]
      shift-right: [w114] -> w36
      shift-left: w35 -> [w114]
      tunnel: w25 -> [w113]
      tunnel: [w112] -> w23
      shift-right: [w110] -> w21
      shift-left: w22 -> [w111]
      shift-right: [w104] -> w18
      shift-left: w19 -> [w105]
      stop <- TRUE stop-if-true
      n15 = case shown="\"minus two\"" w113 {
        selector: w113 -> [w133 w160 w171 w210 w254 w277 w338 w388]
        tunnel: w122 -> [w138 w159 w178 w217 w246 w281 w344 w395]
        tunnel: w121 -> [w134 w156 w177 w216 w244 w280 w343 w394]
        tunnel: w120 -> [w140 w157 w176 w215 w241 w279 w342 w393]
        tunnel: [w139 w157 w175 w214 w241 w263 w329 w392] -> w119
        tunnel: [w135 w158 w174 w213 w240 w272 w341 w391] -> w118
        tunnel: [w136 w159 w173 w212 w245 w273 w340 w390] -> w117
        tunnel: w116 -> [w137 w158 w172 w211 w240 w278 w339 w389]
        tunnel: [w128 w156 w164 w203 w248 w266 w334 w377] -> w108
        tunnel: [w133 w160 w171 w210 w254 w277 w338 w388] -> w112
        tunnel: [w132 w155 w170 w209 w253 w276 w337 w384] -> w110
        tunnel: w111 -> [w132 w155 w170 w209 w253 w276 w337 w385]
        tunnel: [w127 FALSE w163 w202 w247 w268 w330 w376] -> w109
        tunnel: w107 -> [w124 w154 w166 w205 w249 w265 w332 w380]
        tunnel: [w125 w154 w167 w206 w250 w264 w331 w381] -> w106
        tunnel: w105 -> [w123 w152 w161 w200 w239 w255 w324 w375]
        tunnel: [w123 w152 w161 w199 w239 w255 w324 w375] -> w104
        frame "five" {
          (unwired) 0.0
          n16 = while {
            shift-right: [w141] -> w129
            shift-left: w134 -> [w141]
            shift-right: [w150] -> w126
            shift-left: _ -> [_]
            shift-right: [w145] -> w139
            shift-left: w140 -> [w145]
            shift-right: [w143] -> w136
            shift-left: w138 -> [w143]
            shift-right: [w144] -> w135
            shift-left: w137 -> [w144]
            stop <- TRUE stop-if-true
            n17 = Unbundle By Name(w141) -> ("left"=w148:i32, "window"=w149:i32, "center"=w147:i32)
            n18 = Array Subset(array=w145, index=w148, length=w149) -> (w151:cdb[])
            n19 = Subtract(x=w147, y=w148) -> (x-y=w146:i32)
            n20 = call "linear interpolation iiii- complex.vi"("Array"=w151, "center"=w146) -> ("center"=w150:cdb)  [unwired: 5 in, 8 out]
          }
          n21 = Unbundle By Name(w129) -> ("center"=w130:i32)
          n22 = Replace Array Subset(array=w124, new element=w126, index=w130) -> (w125:cdb[])
          n23 = call "tale of three indices.vi"("selector"=tale_of_three_indices_--_selector_--_control."all right", "tale of three indices -- int -- control"=w129) -> ("at right end?"=w127:bool, "tale of three indices -- int -- control out"=w128:T2)  [unwired: 6 in, 2 out]
        }
        frame "zero", Default {
          (unwired) 0.0
          # "no filter"
        }
        frame "two" {
          n24 = while {
            shift-right: [w185] -> w162
            shift-left: w177 -> [w186]
            shift-right: [w197] -> w165
            shift-left: _ -> [_]
            shift-right: [w192] -> w175
            shift-left: w176 -> [w192]
            shift-right: [w190] -> w173
            shift-left: w178 -> [w190]
            shift-right: [w191] -> w174
            shift-left: w172 -> [w191]
            i -> [w183]
            stop <- w187 stop-if-true
            n25 = Unbundle By Name(w186) -> ("left"=w195:i32, "window"=w196:i32, "center"=w194:i32)
            n26 = Array Subset(array=w192, index=w195, length=w196) -> (w198:cdb[])
            n27 = Subtract(x=w194, y=w195) -> (x-y=w193:i32)
            n28 = Equal To 0?(x=w183) -> (x = 0?=w182:bool)
            n29 = call "linear interpolation - bb - complex.vi"("Array"=w198, "center"=w193) -> ("bb"=w179:dbl, "center"=w197:cdb)  [unwired: 5 in, 7 out]
            n30 = Multiply(x=w190, y=1.01) -> (x*y=w188:dbl)
            n31 = call "Q -- check range -- i -- real.vi"("upper"=w188, "lower"=w190, "number"=w179) -> ("selector"=w184:T4)  [unwired: 6 in, 2 out]
            n32 = call "filter -- window span logic.vi"("action for \"above\""=tale_of_three_indices_--_selector_--_control."shrink" ("selector"), "action for \"below\""=tale_of_three_indices_--_selector_--_control."grow" ("selector"), "tale of three indices -- int -- control out"=w186, "start"=w182, "new state"=w184) -> ("three indices out"=w185:T2, "stop"=w187:bool)  [unwired: 5 in]
          }
          n33 = Unbundle By Name(w162) -> ("center"=w168:i32)
          n34 = Replace Array Subset(array=w166, new element=w165, index=w168) -> (w167:cdb[])
          n35 = call "tale of three indices.vi"("selector"=tale_of_three_indices_--_selector_--_control."all right", "tale of three indices -- int -- control"=w162) -> ("at right end?"=w163:bool, "tale of three indices -- int -- control out"=w164:T2)  [unwired: 6 in, 2 out]
        }
        frame "minus two" {
          n36 = while {
            shift-right: [w225] -> w201
            shift-left: w216 -> [w226]
            shift-right: [w237] -> w204
            shift-left: _ -> [_]
            shift-right: [w232] -> w214
            shift-left: w215 -> [w232]
            shift-right: [w230] -> w212
            shift-left: w217 -> [w230]
            shift-right: [w231] -> w213
            shift-left: w211 -> [w231]
            shift-right: [w218] -> w199
            shift-left: w200 -> [w218]
            i -> [w223]
            stop <- w227 stop-if-true
            n37 = Unbundle By Name(w226) -> ("left"=w235:i32, "window"=w236:i32, "center"=w234:i32)
            n38 = Array Subset(array=w232, index=w235, length=w236) -> (w238:cdb[])
            n39 = Subtract(x=w234, y=w235) -> (x-y=w233:i32)
            n40 = Equal To 0?(x=w223) -> (x = 0?=w222:bool)
            n41 = call "linear interpolation - bb - complex.vi"("Array"=w238, "center"=w233) -> ("bb"=w219:dbl, "center"=w237:cdb)  [unwired: 5 in, 7 out]
            n42 = Multiply(x=w230, y=1.01) -> (x*y=w228:dbl)
            n43 = call "Q -- check range -- i -- real.vi"("upper"=w228, "lower"=w230, "number"=w219) -> ("selector"=w224:T4)  [unwired: 6 in, 2 out]
            n44 = call "filter -- window span logic.vi"("action for \"above\""=tale_of_three_indices_--_selector_--_control."shrink" ("selector"), "action for \"below\""=tale_of_three_indices_--_selector_--_control."grow" ("selector"), "tale of three indices -- int -- control out"=w226, "start"=w222, "new state"=w224) -> ("three indices out"=w225:T2, "stop"=w227:bool)  [unwired: 5 in]
          }
          n45 = Unbundle By Name(w201) -> ("center"=w207:i32)
          n46 = Replace Array Subset(array=w205, new element=w204, index=w207) -> (w206:cdb[])
          n47 = call "tale of three indices.vi"("selector"=tale_of_three_indices_--_selector_--_control."all right", "tale of three indices -- int -- control"=w201) -> ("at right end?"=w202:bool, "tale of three indices -- int -- control out"=w203:T2)  [unwired: 6 in, 2 out]
        }
        frame "minus one" {
          n48 = call "filter -- balance logic.vi"("tale of three indices"=w244, "span"=w246, "Array"=w241) -> ("three indices out"=w243:T2, "center out"=w242:cdb, "span out"=w245:dbl)  [unwired: 5 in, 1 out]
          n49 = Unbundle By Name(w243) -> ("center"=w251:i32)
          n50 = Replace Array Subset(array=w249, new element=w242, index=w251) -> (w250:cdb[])
          n51 = call "tale of three indices.vi"("selector"=tale_of_three_indices_--_selector_--_control."center right", "tale of three indices -- int -- control"=w243) -> ("at right end?"=w247:bool, "tale of three indices -- int -- control out"=w248:T2)  [unwired: 6 in, 2 out]
        }
        frame "one" {
          n52 = while {
            shift-right: [w313] -> w270
            shift-left: w280 -> [w314]
            shift-right: [w320] -> w275
            shift-left: w279 -> [w320]
            shift-right: [w318] -> w274
            shift-left: w281 -> [w318]
            shift-right: [w319] -> w271
            shift-left: w278 -> [w319]
            shift-right: [w306] -> w256
            shift-left: _ -> [_]
            i -> [w311]
            stop <- w315 stop-if-true
            n53 = Unbundle By Name(w314) -> ("left"=w322:i32, "center"=w321:i32)  [unwired: 1 out]
            n54 = Subtract(x=w321, y=w322) -> (x-y=w307:i32)
            n55 = Array Subset(array=w320, index=w322, length=w307) -> (w323:cdb[])
            n56 = Equal To 0?(x=w311) -> (x = 0?=w310:bool)
            n57 = call "linear interpolation iiii- complex.vi"("Array"=w323) -> ("directed sigma"=w306:dbl)  [unwired: 6 in, 8 out]
            n58 = Multiply(x=w318, y=1.01) -> (x*y=w316:dbl)
            n59 = call "Q -- check range -- i -- real.vi"("upper"=w316, "lower"=w318, "number"=w306) -> ("selector"=w312:T4)  [unwired: 6 in, 2 out]
            n60 = call "filter -- window span logic.vi"("action for \"above\""=tale_of_three_indices_--_selector_--_control."left wing shrink" ("selector"), "action for \"below\""=tale_of_three_indices_--_selector_--_control."left wing grow" ("selector"), "tale of three indices -- int -- control out"=w314, "start"=w310, "new state"=w312) -> ("three indices out"=w313:T2, "stop"=w315:bool)  [unwired: 5 in]
          }
          n61 = while {
            shift-right: [w300] -> w267
            shift-left: w270 -> [w301]
            shift-right: [w291] -> w263
            shift-left: w275 -> [w291]
            shift-right: [w303] -> w273
            shift-left: w274 -> [w303]
            shift-right: [w304] -> w272
            shift-left: w271 -> [w304]
            shift-right: [w292] -> _
            shift-left: w256 -> [w292]
            i -> [w298]
            stop <- w302 stop-if-true
            n62 = Unbundle By Name(w301) -> ("right"=w294:i32, "left"=w288:i32, "center"=w290:i32)
            n63 = Subtract(x=w294, y=w290) -> (x-y=w293:i32)
            n64 = Subtract(x=w290, y=w288) -> (x-y=w289:i32)
            n65 = Equal To 0?(x=w298) -> (x = 0?=w297:bool)
            n66 = Array Subset(array=w291, index=w288, length=w289) -> (w287:cdb[])
            n67 = Array Subset(array=w291, index=w290, length=w293) -> (w305:cdb[])
            n68 = call "linear interpolation iiii- complex.vi"("Array"=w287) -> ("directed sigma"=w285:dbl)  [unwired: 6 in, 8 out]
            n69 = call "linear interpolation iiii- complex.vi"("Array"=w305) -> ("directed sigma"=w286:dbl)  [unwired: 6 in, 8 out]
            n70 = Subtract(x=w286, y=w285) -> (x-y=w284:dbl)
            n71 = call "Q -- check range -- i -- real.vi"("upper"=0.001 ("y"), "lower"=-0.001 ("y"), "number"=w284) -> ("selector"=w299:T4)  [unwired: 6 in, 2 out]
            n72 = call "filter -- window span logic.vi"("action for \"above\""=tale_of_three_indices_--_selector_--_control."window left" ("selector"), "action for \"below\""=tale_of_three_indices_--_selector_--_control."window right" ("selector"), "tale of three indices -- int -- control out"=w301, "start"=w297, "new state"=w299) -> ("three indices out"=w300:T2, "stop"=w302:bool)  [unwired: 5 in]
          }
          n73 = Unbundle By Name(w267) -> ("left"=w259:i32, "window"=w262:i32, "center"=w260:i32)
          n74 = Array Subset(array=w263, index=w259, length=w262) -> (w261:cdb[])
          n75 = call "tale of three indices.vi"("selector"=tale_of_three_indices_--_selector_--_control."center right", "tale of three indices -- int -- control"=w267) -> ("no success ?"=w268:bool, "tale of three indices -- int -- control out"=w266:T2)  [unwired: 6 in, 2 out]
          n76 = Subtract(x=w260, y=w259) -> (x-y=w258:i32)
          n77 = call "linear interpolation iiii- complex.vi"("Array"=w261, "center"=w258) -> ("center"=w257:cdb)  [unwired: 5 in, 8 out]
          n78 = Replace Array Subset(array=w265, new element=w257, index=w260) -> (w264:cdb[])
        }
        frame "four" {
          (unwired) 0.0
          n79 = while {
            shift-right: [w370] -> w333
            shift-left: w343 -> [w371]
            shift-right: [w362] -> w329
            shift-left: w342 -> [w362]
            shift-right: [w350] -> w340
            shift-left: w344 -> [w350]
            shift-right: [w372] -> w341
            shift-left: w339 -> [w372]
            i -> [w367]
            stop <- w369 stop-if-true
            w347 = tale_of_three_indices_--_selector_--_control."shrink"  # action for "above"
            w348 = tale_of_three_indices_--_selector_--_control."grow"  # action for "below"
            (unwired) 1.01 ("y")
            n80 = Unbundle By Name(w371) -> ("left"=w373:i32, "right"=w361:i32, "center"=w360:i32)
            n81 = Subtract(x=w360, y=w373) -> (x-y=w365:i32)
            n82 = Subtract(x=w361, y=w360) -> (x-y=w363:i32)
            n83 = Array Subset(array=w362, index=w373, length=w365) -> (w374:cdb[])
            n84 = Array Subset(array=w362, index=w360, length=w363) -> (w364:cdb[])
            n85 = call "linear interpolation iiii- complex.vi"("Array"=w374, "center"=w365) -> ("slope"=w358:cdb)  [unwired: 5 in, 8 out]
            n86 = call "linear interpolation iiii- complex.vi"("Array"=w364, "center"=w363) -> ("slope"=w356:cdb)  [unwired: 5 in, 8 out]
            n87 = Complex To Polar(r * e^(i*theta)=w356) -> (r=w357:dbl)  [unwired: 1 out]
            n88 = Equal To 0?(x=w367) -> (x = 0?=w366:bool)
            n89 = Complex To Polar(r * e^(i*theta)=w358) -> (r=w359:dbl)  [unwired: 1 out]
            n90 = Divide(x=w356, y=w357) -> (x/y=w355:cdb)
            n91 = Divide(x=w358, y=w359) -> (x/y=w353:cdb)
            n92 = Complex Conjugate(1:w355) -> (0:w354:cdb)
            n93 = Multiply(x=w353, y=w354) -> (x*y=w352:cdb)
            n94 = Complex To Re/Im(x + iy=w352) -> (y=w351:dbl)  [unwired: 1 out]
            n95 = Absolute Value(x=w351) -> (abs(x)=w349:dbl)
            n96 = call "Q -- check range -- i -- real.vi"("upper"=0.1 ("y"), "lower"=0.05 ("y"), "number"=w349) -> ("selector"=w368:T4)  [unwired: 6 in, 2 out]
            n97 = call "filter -- window span logic.vi"("action for \"above\""=w347, "action for \"below\""=w348, "tale of three indices -- int -- control out"=w371, "start"=w366, "new state"=w368) -> ("three indices out"=w370:T2, "stop"=w369:bool)  [unwired: 5 in]
          }
          n98 = Unbundle By Name(w333) -> ("left"=w326:i32, "window"=w325:i32, "center"=w335:i32)
          n99 = Array Subset(array=w329, index=w326, length=w325) -> (w328:cdb[])
          n100 = call "tale of three indices.vi"("selector"=tale_of_three_indices_--_selector_--_control."all right", "tale of three indices -- int -- control"=w333) -> ("at right end?"=w330:bool, "tale of three indices -- int -- control out"=w334:T2)  [unwired: 6 in, 2 out]
          n101 = call "linear interpolation iiii- complex.vi"("Array"=w328) -> ("center"=w327:cdb)  [unwired: 6 in, 8 out]
          n102 = Replace Array Subset(array=w332, new element=w327, index=w335) -> (w331:cdb[])
        }
        frame "three" {
          n103 = while {
            shift-right: [w424] -> w378
            shift-left: w394 -> [w423]
            shift-right: [w399] -> w379
            shift-left: _ -> [_]
            shift-right: [w420] -> w392
            shift-left: w393 -> [w420]
            shift-right: [w418] -> w390
            shift-left: w395 -> [w418]
            shift-right: [w419] -> w391
            shift-left: w389 -> [w419]
            shift-right: [w413] -> _
            shift-left: comparison_control."not a number" ("selector") -> [w415]
            shift-right: [w412] -> _
            shift-left: 0 -> [w414]
            shift-right: [w398] -> w384
            shift-left: w385 -> [w405]
            i -> [w407]
            stop <- w408 stop-if-true
            n104 = Unbundle By Name(w423) -> ("left"=w404:i32, "window"=w422:i32, "center"=w406:i32)
            n105 = Subtract(x=w406, y=w404) -> (x-y=w402:i32)
            n106 = Array Subset(array=w420, index=w404, length=w422) -> (w426:cdb[])
            n107 = Multiply(x=w418, y=1.01) -> (x*y=w416:dbl)
            n108 = call "linear interpolation iiii- complex.vi"("Array"=w426, "center"=w402) -> ("directed sigma"=w421:dbl, "intercept"=w400:cdb, "slope"=w397:cdb)  [unwired: 5 in, 6 out]
            n109 = call "Q -- check range -- i -- real.vi"("upper"=w416, "lower"=w418, "number"=w421) -> ("selector"=w425:T4)  [unwired: 6 in, 2 out]
            n110 = case shown="\"above\"" w425 {
              selector: w425 -> [_ w432 w446]
              tunnel: [TRUE w431 w445] -> w410
              tunnel: [w430 w438 w451] -> w424
              tunnel: w423 -> [w430 w439 w452]
              tunnel: w415 -> [w428 w436 w450]
              tunnel: [w427 w435 w448] -> w412
              tunnel: w414 -> [w427 w434 w449]
              tunnel: [w428 w433 w447] -> w413
              frame "in range", Default {
              }
              frame "above" {
                n111 = call "tale of three indices.vi"("selector"=tale_of_three_indices_--_selector_--_control."shrink", "tale of three indices -- int -- control"=w439) -> ("no success ?"=w431:bool, "tale of three indices -- int -- control out"=w438:T2)  [unwired: 6 in, 2 out]
                n112 = case shown="\"below\"" w436 {
                  tunnel: [w440 w442] -> w435
                  tunnel: w434 -> [w440 w443]
                  tunnel: [w441 w444] -> w433
                  tunnel: w432 -> [w441 w444]
                  frame "not a number", Default {
                  }
                  frame "below" {
                    n113 = Increment(x=w443) -> (x+1=w442:i32)
                  }
                }
              }
              frame "below" {
                n114 = case shown="\"above\"" w450 {
                  tunnel: [w454 w456] -> w448
                  tunnel: w449 -> [w454 w457]
                  tunnel: [w455 w458] -> w447
                  tunnel: w446 -> [w455 w458]
                  frame "not a number", Default {
                  }
                  frame "above" {
                    n115 = Increment(x=w457) -> (x+1=w456:i32)
                  }
                }
                n116 = call "tale of three indices.vi"("selector"=tale_of_three_indices_--_selector_--_control."grow", "tale of three indices -- int -- control"=w452) -> ("no success ?"=w445:bool, "tale of three indices -- int -- control out"=w451:T2)  [unwired: 6 in, 2 out]
              }
            }
            n117 = Replace Array Subset(array=w405, new element=w397, index=w406) -> (w398:cdb[])
            n118 = Array Subset(array=w398, index=w404, length=w402) -> (w403:cdb[])
            n119 = call "linear interpolation iiii- complex.vi"("Array"=w403, "center"=w402) -> ("interpolated average"=w396:cdb)  [unwired: 5 in, 8 out]
            n120 = Multiply(x=w396, y=w402) -> (x*y=w401:cdb)
            n121 = Greater?(x=w412, y=3) -> (0:w409:bool)
            n122 = Or(x=w410, y=w409) -> (x .or. y?=w408:bool)
            n123 = Add(x=w400, y=w401) -> (x+y=w399:cdb)
            "Numeric 2" <- w407
          }
          n124 = Unbundle By Name(w378) -> ("center"=w382:i32)
          n125 = Replace Array Subset(array=w380, new element=w379, index=w382) -> (w381:cdb[])
          n126 = call "tale of three indices.vi"("selector"=tale_of_three_indices_--_selector_--_control."all right", "tale of three indices -- int -- control"=w378) -> ("at right end?"=w376:bool, "tale of three indices -- int -- control out"=w377:T2)  [unwired: 6 in, 2 out]
        }
      }
    }
    n127 = Or(x=w37, y=w26) -> (x .or. y?=w32:bool)
  }
  "omega out" <- w1
  "center" <- w10
  "norm" <- w11
  "at right end?" <- w16
  "tale of three indices -- int -- control out" <- w9
  "z in out" <- w3
  n128 = Multiply(x=w11, y=w12) -> (x*y=w13:cdb[])
  n129 = Add(x=w13, y=w10) -> (x+y=→"z out":cdb[])
